vi "HostMain.vi"() -> ()   [LabVIEW 2024]
uses:
  C:/Users/ROAR/Documents/Darren RobUST/grf-mpc-RobUST-trainer/Labview/RobUST_3D_with_Unity_Control_PXI_Low_Level_Only_Streamlined/Vicon_files/ViconDataStreamSDK_DotNET.dll
  Vicon_files/ViconDataStreamSDK_DotNET.dll
  typeDef/Modes_knees.ctl
  <vilib>/Platform/TimedLoop/XDataNode/timing_clust.ctl
  <vilib>/Platform/TimedLoop/XDataNode/nitl_modes.ctl
  <vilib>/Platform/TimedLoop/XDataNode/wakeup.ctl
  <vilib>/Utility/file.llb/Read Delimited Spreadsheet (DBL).vi
  <vilib>/platform/TimedLoop/XDataNode/XDataNode.xnode
  <vilib>/Utility/Variable/NI_VariableUtilities.lvlib
  <vilib>/Platform/TimedLoop/XDataNode/XDNodeRunTimeDep.lvlib
  <vilib>/Analysis/NI_AALBase.lvlib
panel:
  out "listener ID":refnum<k5>
  out "Tokenized Unity Message":string[](array[string])
  out "All tensions mean":dbl[](array[numeric])
  out "Captured tensions mean":dbl[](array[numeric])
  out "Captured tensions standard dev":dbl[](array[numeric])
  in  "Capture current tension mean and standard dev":bool
  out "All tensions standard dev":dbl[](array[numeric])
  out "All tensions history":dbl[][](array[numeric])
  in  "ConstantModeActiveMotorFlags":bool[](array[boolean])
  out "StartManualTensionRecordTimeInSeconds":dbl
  out "RecordTime (s)":dbl
  out "Manually record tensions flag previous state":bool
  in  "MaxTensionsRecordTimeInSecs":dbl
  in  "RecordTensionsForGivenTimeFlag":bool
  out "Task has ended flag":bool
  out "Tension tare values":dbl[](array[numeric])
  in  "Live plot tensions flag":bool
  out "New info string received":bool
  out "Unity task info string":string
  in  "Use sinusoid":bool
  in  "Sinusoid period (s)":dbl
  in  "Sinusoid amplitude (N)":dbl
  in  "Single motor number":i32
  in  "Single motor tension current set value":dbl=10.0 min=10.0
  in  "Single motor tension desired set value":dbl
  in  "Change constant tension value toggle":bool
  out "Finished Late? [i-1]":bool
  out "CablesTared?":bool
  out "Data to save":dbl[][](array[numeric])
  out "Current save file out":path
  out "Connected to Unity last save call?":bool
  in  "Constant mode cable tensions N":dbl
  out "Last Vicon Frame Read":u32
  out "LastTimeUnityTensionsReceivedInMs":u32
  out "TensionsUpdateRateHz":dbl
  out "UnityDesiredCableTensionsInAscendingOrder":dbl[](array[numeric])
  in  "Mode Robot":T1(radio)
  in  "Total Number Motors":i32
  out "Latest tensions":dbl[](array[numeric])
  in  "Tare":bool
  out "Trunk Structure Matrix":dbl[][](array[numeric])
  out "Trunk FF type specifier":string
  out "Center point for FF":dbl[](array[numeric])
  out "Excursion distances Vicon frame":dbl[](array[numeric])
  out "TCP connection to Unity?":bool
  out "Unity TCP connection ID":refnum<k5>
  out "Control point position coords":dbl[](array[numeric])
  in  "Control point data source":T2(radio)
  in  "perturbation directions":string
  in  "Refresh Center 2":bool
  in  "Insert Test Name":string
  out "CurrentPttrunk":cluster{dbl[], dbl[]}
  out "Centertrunk":cluster{dbl[], dbl[]}
  out "xyboundstrunk":cluster{dbl[], dbl[]}
  out "trunk markers":dbl[](array[numeric])
  out "pel markers":dbl[](array[numeric])
  out "whichMode 3":bool[](array[boolean])
  in  "Mode Knees":T3
  out "whichMode 2":bool[](array[boolean])
  in  "?":enum32{"Trunk FF", "Pelvis FF"}(tab)
  in  "Turn On":bool
  out "Trunk Graph":cluster{dbl[], dbl[]}[](graph)
  out "Pelvis Graph":cluster{dbl[], dbl[]}[](graph)
  in  "Turn On Pelv":bool
  out "PelvisGraphyz":cluster{dbl[], dbl[]}[](graph)
  in  "?":T4(tab)
  in  "% Body Weight":dbl=10.0
  in  "FM --- FF":dbl[](array[numeric])=[30.0, 15.0, 15.0, 15.0, 2.0, 2.0]
  in  "Force Field Radius (m)":dbl=0.05
  in  "Update R or FF":bool
  in  "Refresh Center":bool
  in  "Select File with Trunk\nBoundary Points":path=path "" caption="start path"
  in  "Pert Reset":bool
  in  "Apply Pert":bool
  out "Weight [lbs]":dbl
  in  "Update Pert Parameters":bool
  in  "Pert Direction":i16(knob) scale=0.0..7.0
  in  "Rise Time":dbl
  in  "Constant Time":dbl
  in  "Fall Time":dbl
  in  "Amp [%BW]":dbl
  in  "Weight [Kg]":dbl
  in  "Mode Pelvis":enum32{"Idle", "Constant", "Force", "Pert"}(radio)
  out "Boolean":bool
  out "14":cluster{"[0]":dbl, "[1]":dbl}(graph)
  out "13":cluster{"[0]":dbl, "[1]":dbl}(graph)
  out "12":cluster{"[0]":dbl, "[1]":dbl}(graph)
  out "11":cluster{"[0]":dbl, "[1]":dbl}(graph)
  out "10":cluster{"[0]":dbl, "[1]":dbl}(graph)
  out "9":cluster{"[0]":dbl, "[1]":dbl}(graph)
  in  "?":T5(tab)
  in  "Reset Label":bool
  out "Going Up":bool
  in  "record trajectory":bool
  in  "Weight (Kg) --- FF 2":dbl=50.0
  in  "% Body Weight 2":dbl=10.0
  in  "FM --- FF 2":dbl[](array[numeric])=[30.0, 5.0, 5.0, 5.0, 2.0, 2.0]
  in  "Update R or FF 2":bool
  in  "Pelvis Radius FF":dbl=0.03
  in  "Weight [Kg] 3":dbl=75.0
  in  "Amp [%BW] 3":dbl=10.0
  in  "Fall Time 2":dbl=200.0
  in  "Constant Time 2":dbl=200.0
  in  "Rise Time 2":dbl=200.0
  in  "Pert Direction 2":i16(knob) scale=0.0..7.0
  in  "Update Pert Parameters 2":bool
  out "Weight [lbs] 3":dbl
  in  "Apply Pert 2":bool
  in  "Pert Reset 2":bool
  in  "Set Unit Force Vector":dbl[](array[numeric])=[0.0, 0.0, -1.0, 15.0, 2.0, 2.0]
  in  "Update_setForces":bool
  in  "Set % Body Weight":dbl=10.0
  in  "Weight (lb)":dbl=50.0
  out "ATI":dbl[](graph)
  in  "ATI UnBias":bool
  in  "ATI Bias":bool
  out "Saving Data":bool
  out "whichMode":bool[](array[boolean])
  in  "pidGains":dbl[][](array[numeric])=[[3.5, 1.7, 3.0000000000000004, 1.7, 1.7, 3.5, 1.7, 1.7, 2.0, 1.7, 1.7, 3.0, 1.7, 3.5], [0.001, 0.003, 0.003, 0.001, 0.001, 0.003, 0.0008, 0.003, 0.001, 0.003, 0.001, 0.003, 0.001, 0.001], [0.0004, 0.0012, 0.0006, 0.0012, 0.0012, 0.0004, 0.0012, 0.0012, 0.0008, 0.0012, 0.0012, 0.0004, 0.0012, 0.0004]]
  in  "SetPID":bool
  out "4":cluster{"[0]":dbl, "[1]":dbl}(graph)
  out "3":cluster{"[0]":dbl, "[1]":dbl}(graph)
  out "2":cluster{"[0]":dbl, "[1]":dbl}(graph)
  out "1":cluster{"[0]":dbl, "[1]":dbl}(graph)
  out "8":cluster{"[0]":dbl, "[1]":dbl}(graph)
  out "7":cluster{"[0]":dbl, "[1]":dbl}(graph)
  out "6":cluster{"[0]":dbl, "[1]":dbl}(graph)
  out "FB n FF O/P(N)":dbl[](graph)
  out "Current Filename":string
  out ".NET Reference out":refnum<k24>
  out "ViconTab":enum32{"Vicon", "no Vicon"}(tab)
  out "Frame Number":dbl format="%.2f"
  out "Subject Name":string
  out "Markers Count":u32
  in  "Connect\nVicon":bool
  in  "Update\nMarkers":bool
  in  "Vicon Static":bool
  in  "Stream Mode":i32(ring) items=["ClientPull", "ClientPullPreFetch", "ServerPush"]
  out "SDK Version":string
  out "Vicon Connected":bool
  out "5":cluster{"[0]":dbl, "[1]":dbl}(graph)
  out "Voltage O/P (V)":dbl[](graph)
  in  "Use ATI":bool
  in  "ATIDAQFT._FTSensor":refnum<k7>
  in  "UseVicon":bool
  out "Loop Durations (uSec)":i64[](array[numeric])
  in  "DataSave":bool
  in  "Stop":bool
  # "Notes on running HostMain.vi\n1.)  Start  HostMain (auto in Unity control point mode, Idle Trunk mode).\n2.) Then start targetController.vi (for now)\n3.) The tension sensors MUST be tared when the trunk is in  Idle mode.\n4.) Live tension sensor plots are directly below this text! (scroll down)"
  # "STAND TRAINER\n                     Software developed by Vineet Vashista (2014), Moiz Khan (2016-19), Tatiana Luna (2019-20)"
  # "Unity Communication Info Panel"
  # "TCP Connection Status"
  # "General Robot Constants\n(Set in code)"
  # "Current Unity task information string"
  # "Pelvis-Planar"
  # "Data received from Unity (old, deprecated, could delete!)"
  # "Key coordinates"
  # "----->"
  # "Tare tension sensors panel\nNOTE: tare only works in \nRobotMode = Idle"
  # "Manually start tension recording\n(Note: auto-start with Unity messages\nis typical)"
  # "Robot control panel"
  # "2                          3                                           4                                  5                                      6                        7                                  8                           9                                    10                               11                            12                              13                                   14"
  # "HAVE TO TARE\nBEFORE ROBOT\nMODES BECOME\nENABLED!"
  # "Excursion distance measurements"
  # "Constant mode control"
  # "Single motor mode step change"
  # "Motor 1"
  # "Motor 2"
  # "Motor 3"
  # "Motor 4"
  # "Motor 5"
  # "Motor 6"
  # "Motor 7"
  # "Motor 8"
  # "Motor 9"
  # "FF mode type specifier"
  # "Motor 10"
  # "Types: \"I\" = idle; \"B\" = excursion \nboundary 2D"
  # "Motor 11"
  # "Motor 12"
  # "Motor 13"
  # "Motor 14"
  # "PELVIS TOP MOTORS"
  # "TRUNK MOTOR CABLE \nTENSIONS [N]"
  # "Sensor ID: FT5769"
  # "Mx(Nm)"
  # "My(Nm)"
  # "Mz(Nm)"
  # "PID                   QP                  File"
  # "This can be changed only starting of host"
  # "Pelvis-Moments"
  # "PELVIS BOTTOM MOTORS"
  # "SHANK MOTOR CABLE TENSIONS [N]"
  # "Circular Force Field"
  # "Irregular Force Field"
  # "Fz\nMx\nMy\nMz"
  # "30,15,15,15"
  # "Pert Parameters"
  # "FIRST PERT GIVEN BY\nCLICKING TURN ON PERT!!!"
  # "Pert Parameters"
  # "FIRST PERT GIVEN BY\nCLICKING TURN ON PERT!!!"
  # "X\n\nY\n\nZ"
  # "Trunk Static"
  # "Pelvis Static"
  # "Set Tension = Mag + Constant Tension + Step"
  # "TRUNK CONTROL"
  # "PELVIS CONTROL"
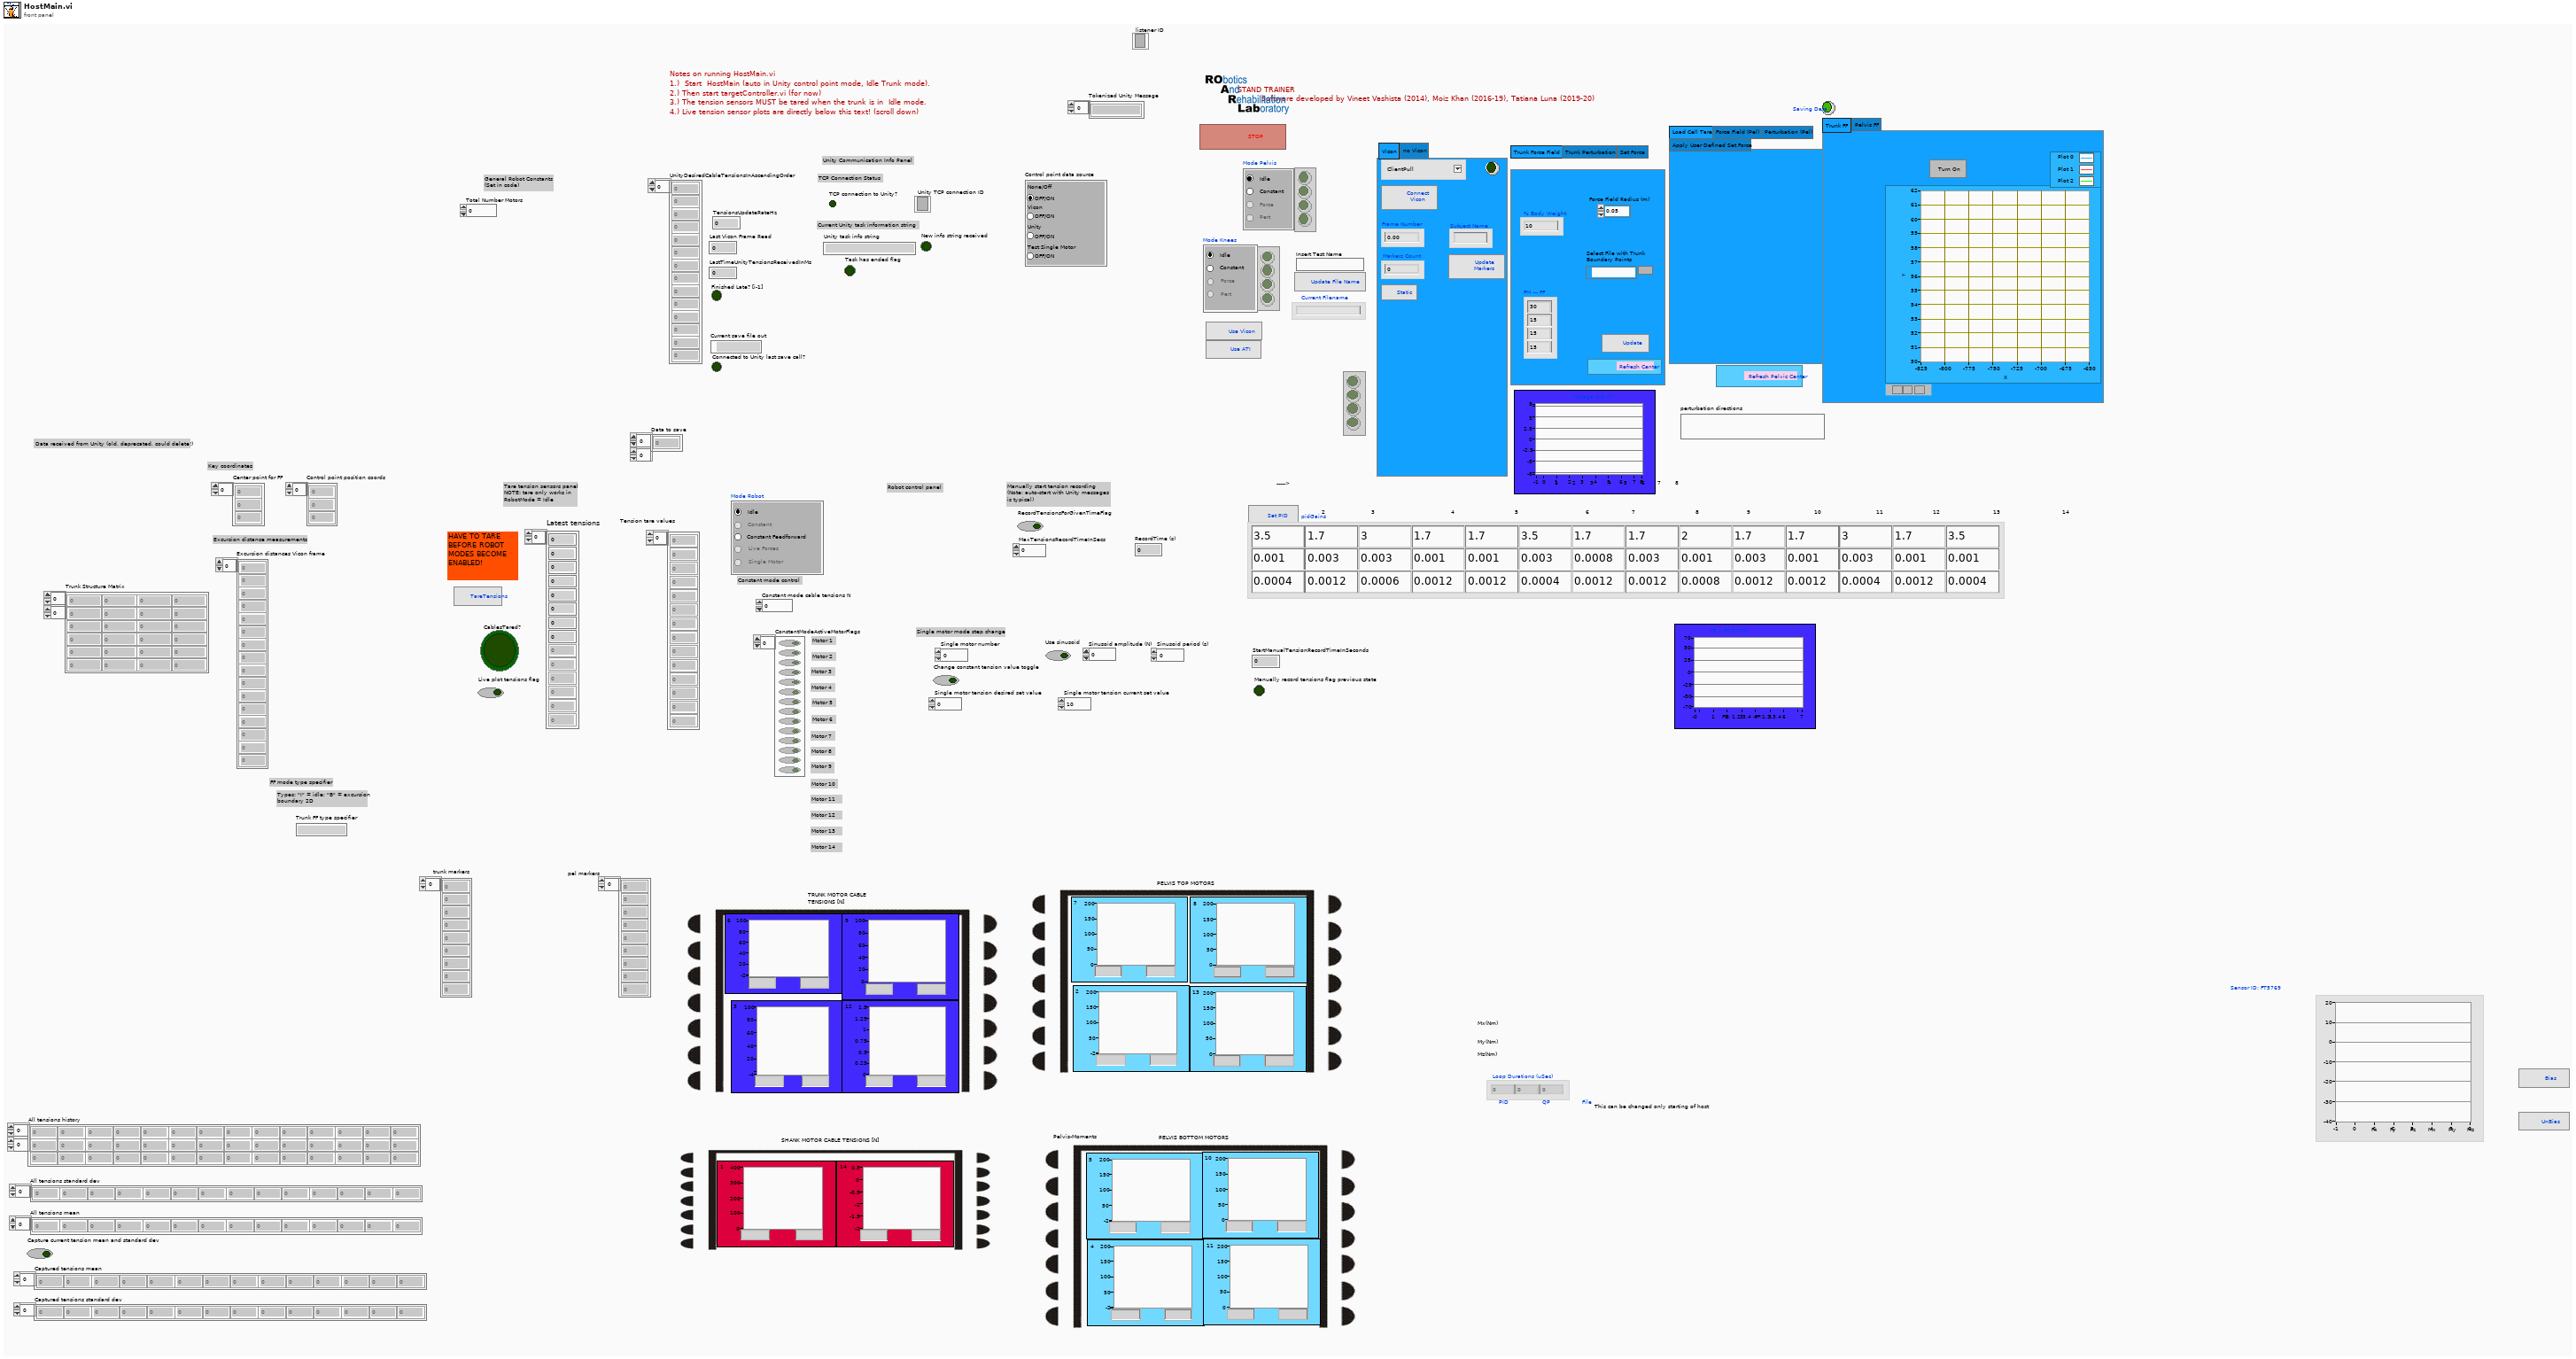
[diagram p1: front panel]
types:
  T1 = enum32{"Idle", "Constant", "Live Forces", "Single Motor", "Constant Feedforward"}
  T2 = enum32{"None/Off", "Vicon", "Unity", "Test Single Motor"}
  T3 = typedef "Modes_knees.ctl" = enum32{"Idle", "Constant", "Force", "Pert"}
  T4 = enum32{"Trunk Force Field", "Trunk Perturbation", "Set Force"}
  T5 = enum32{"Load Cell Tare", "Force Field (Pel)", "Perturbation (Pel)", "Apply User Defined Set Force"}
  T6 = enum32{"Idle", "Constant", "Live Forces", "Single Motor"}
  T7 = enum8{"Enabled", "Disabled", "Disabled and Grayed Out"}
  T8 = typedef "XDNodeRunTimeDep.lvlib/timing_clust.ctl" = cluster{"Expected End [f-1]":u64, "Actual End [f-1]":u64, "Finished Late? [f-1]":bool, "Expected End [i-1]":u64, "Actual End [i-1]":u64, "Finished Late? [i-1]":bool, "Expected Start [i]":u64, "Actual Start [i]":u64, "Expected Start [f]":u64, "Actual Start [f]":u64, "Source Name":string, "Structure Name":string, "Period":i64, "Deadline":i64, "Offset":i64, "Start":i64, "Priority":i32, "Timeout":i32, "Mode":T9, "Wakeup Reason":T10, "Error":errorcluster, "Source Type":string, "Secondary Source Type":string, "Global End Time":u64, "Global Start Time":u64, "Frame Duration":u64, "Iteration Duration":u64, "Assigned CPU":i32, "I/O Scan Engine Mode":u32}
  T9 = typedef "XDNodeRunTimeDep.lvlib/nitl_modes.ctl" = enum32{"No Change", "Process missed periods, maintain original phase", "Discard missed periods, maintain original phase", "Process missed periods, ignore original phase", "Discard missed periods, ignore original phase"}
  T10 = typedef "XDNodeRunTimeDep.lvlib/wakeup.ctl" = enum32{"Normal", "Aborted", "Asynchronous wakeup", "Timing source error", "Timed loop error", "Timeout"}
  T11 = enum16{"Standard", "Buffered", "CRLF", "Immediate"}
  T12 = cluster{"Most Recent Vicon Frame Number":u32, "Corresponding motor tensions":dbl[], "Motor numbers":i32[]}
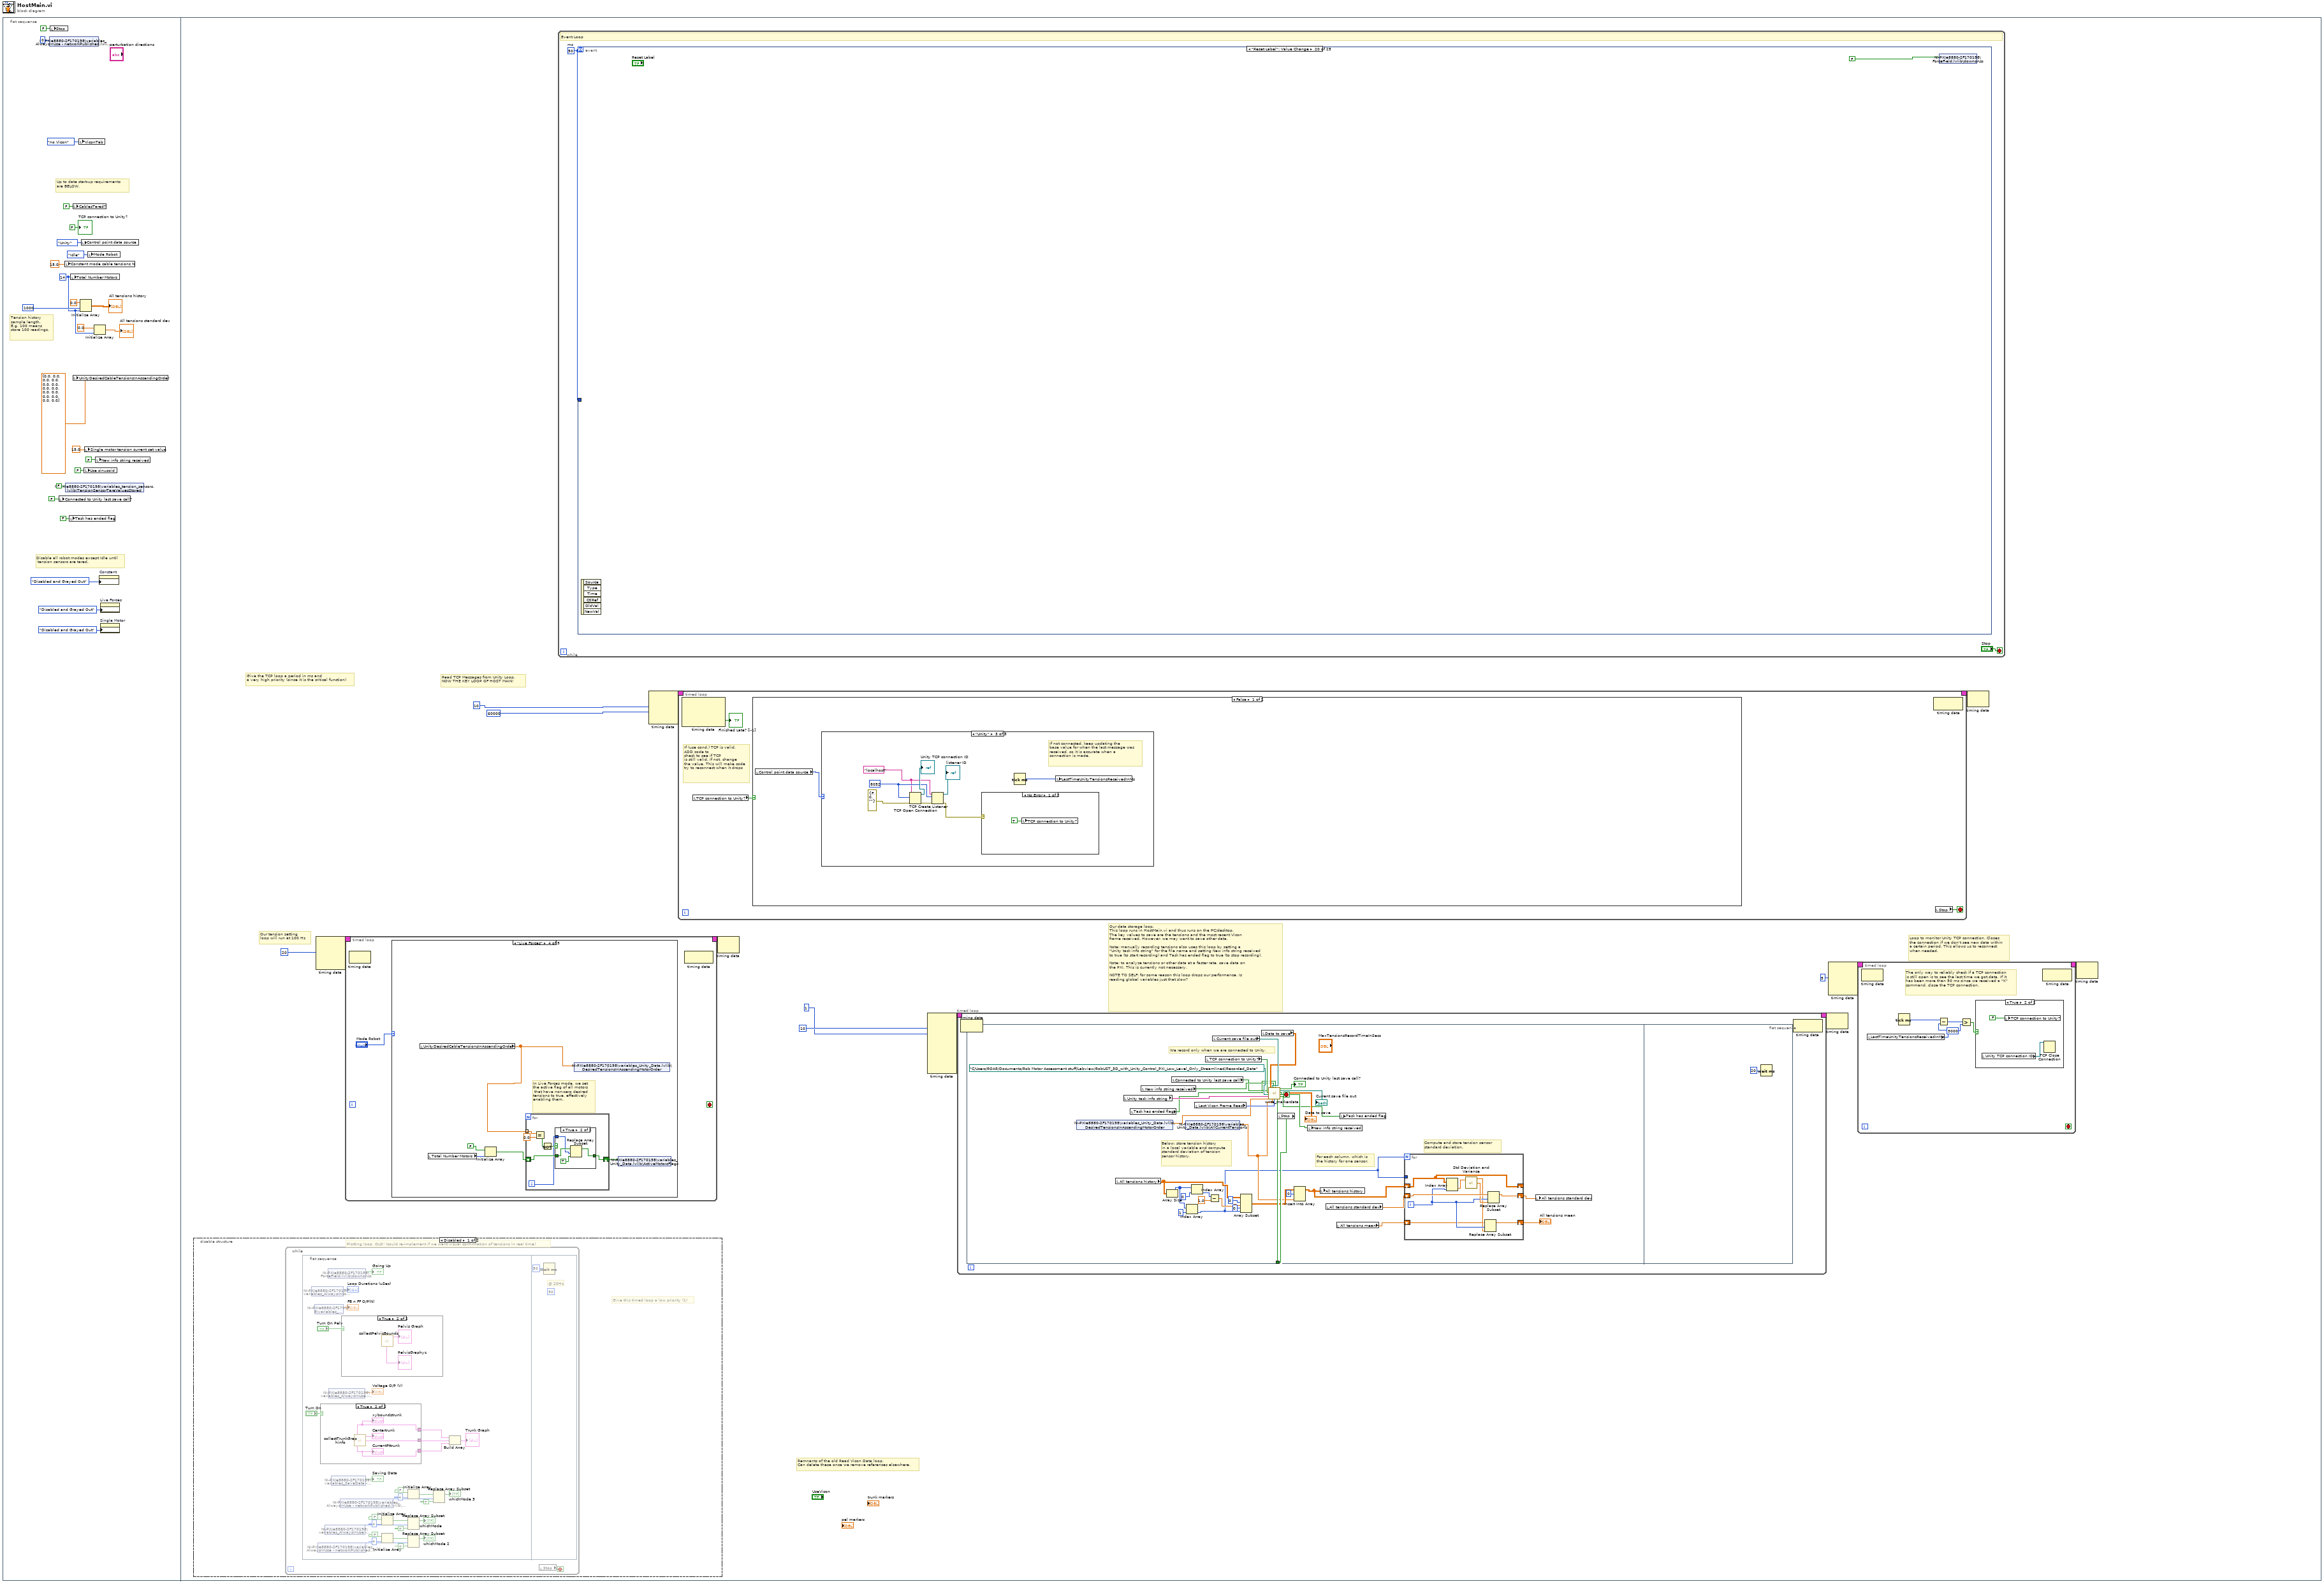
[diagram p0: block diagram]
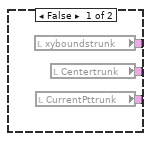
[diagram p3: hidden frame]
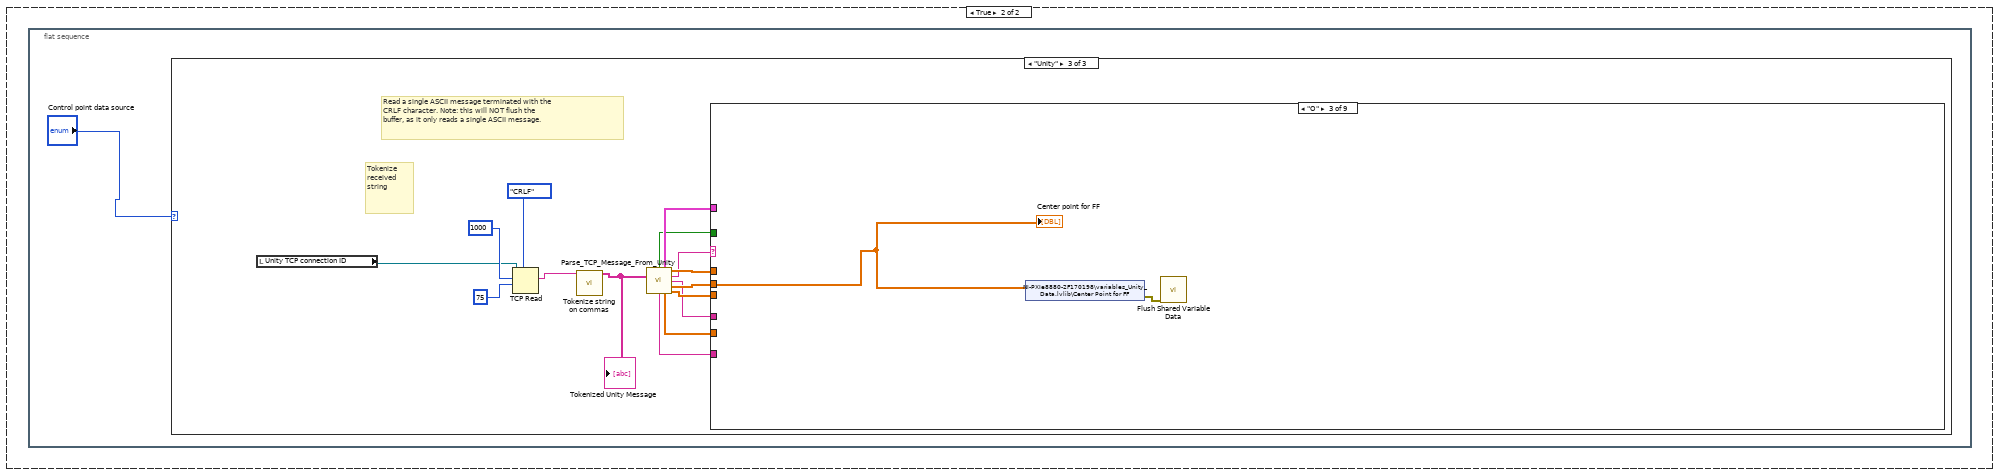
[diagram p9: hidden frame]
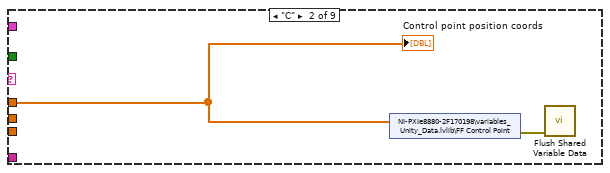
[diagram p13: hidden frame]
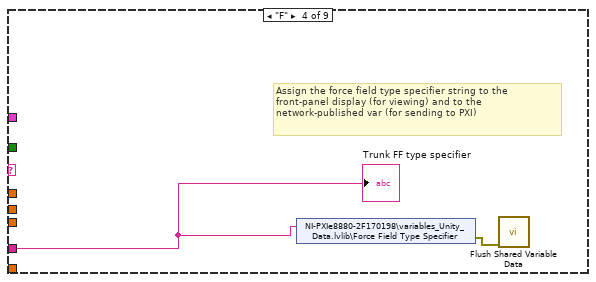
[diagram p14: hidden frame]
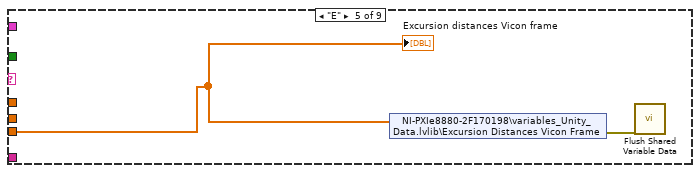
[diagram p15: hidden frame]
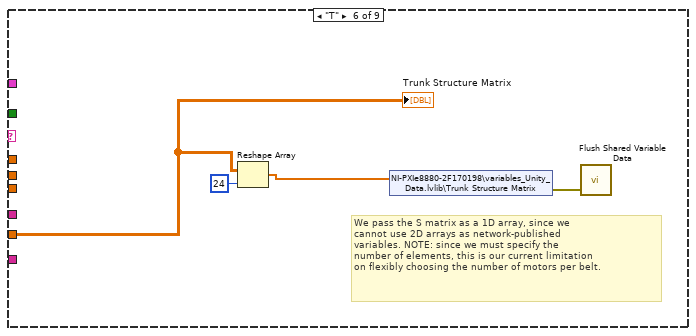
[diagram p16: hidden frame]
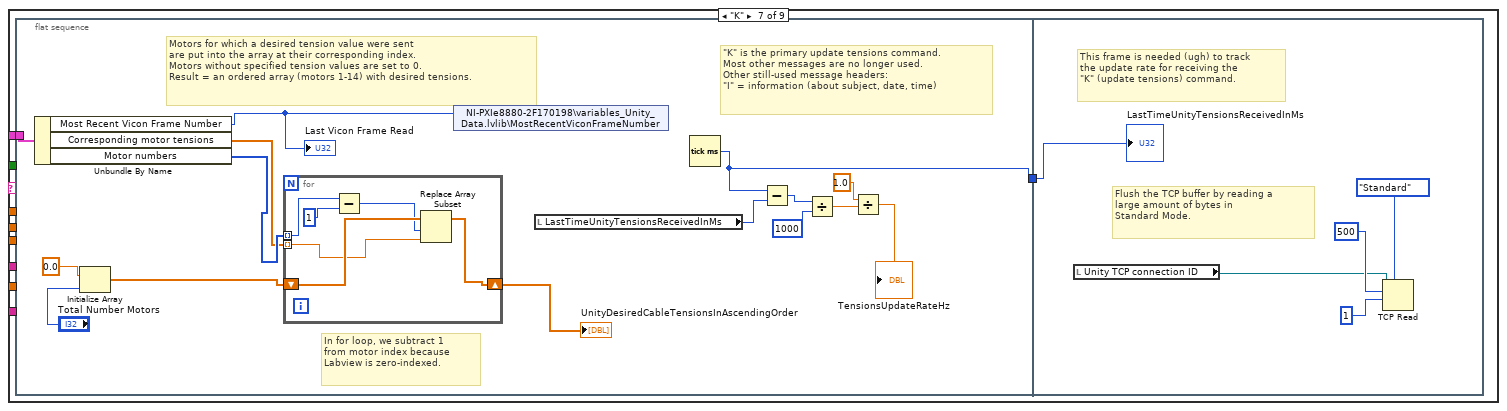
[diagram p17: hidden frame]
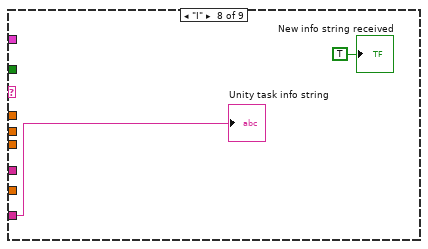
[diagram p18: hidden frame]
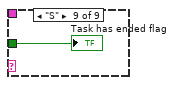
[diagram p19: hidden frame]
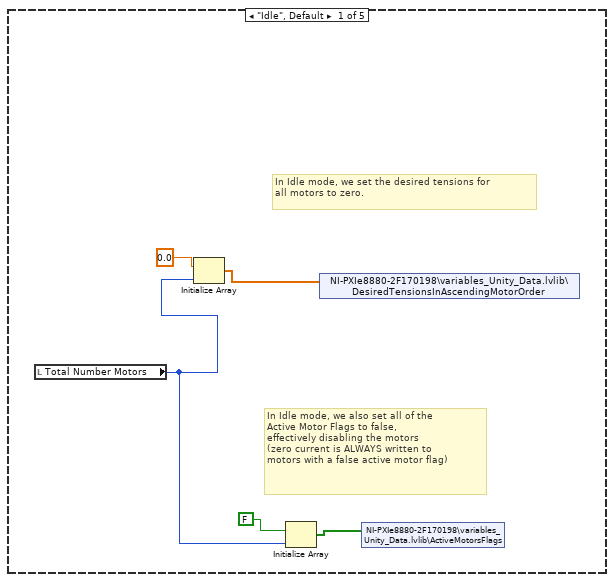
[diagram p20: hidden frame]
diagram:
  n1 = flat-sequence {
    frame #0 {
      w3 = 14 ("Total Number Motors")
      # "Tension history \nsample length. \nE.g. 100 means \nstore 100 readings."
      # "Disable all robot modes except Idle until\n tension sensors are tared."
      # "Up to date start-up requirements\nare BELOW."
      n2 = shared-variable "NI-PXIe8880-2F170198\\variables_AlwaysInUse - networkPublished.lvlib\\Trunk Belt Mode"(i16 0 ("Mode")) -> ()  [unwired: 1 in, 1 out]
      n3 = local write "Stop"(FALSE ("Force")) -> ()
      n4 = local write "Connected to Unity last save call?"(FALSE ("Connected to Unity last save call?")) -> ()
      n5 = local write "Constant mode cable tensions N"(15.0 ("Constant mode cable tensions (N)")) -> ()
      n6 = shared-variable "NI-PXIe8880-2F170198\\variables_tension_sensors.lvlib\\TensionSensorTareValuesStored"(FALSE ("TensionSensorTareValuesStored")) -> ()  [unwired: 1 in, 1 out]
      n7 = local write "Task has ended flag"(FALSE ("Task has ended flag")) -> ()
      n8 = local write "Total Number Motors"(w3) -> ()
      n9 = local write "CablesTared?"(FALSE ("CablesTared?")) -> ()
      n10 = local write "UnityDesiredCableTensionsInAscendingOrder"(dbl[] [0.0, 0.0, 0.0, 0.0, 0.0, 0.0, 0.0, 0.0, 0.0, 0.0, 0.0, 0.0, 0.0, 0.0] ("UnityDesiredCableTensionsInAscendingOrder")) -> ()
      n11 = local write "ViconTab"(enum32{"Vicon", "no Vicon"}."no Vicon" ("ViconTab")) -> ()
      n12 = Initialize Array(0.0 ("element"), 1000 ("dimension size"), w3) -> (→"All tensions history":dbl[][])
      n13 = local write "Control point data source"(enum32{"None/Off", "Vicon", "Unity"}."Unity" ("Control point data source")) -> ()
      n14 = local write "Use sinusoid"(FALSE ("Use sinusoid")) -> ()
      n15 = local write "Single motor tension current set value"(15.0 ("Single motor tension current set value")) -> ()
      n16 = local write "Mode Robot"(T6."Idle" ("Mode Robot")) -> ()
      n17 = Initialize Array(0.0 ("element"), w3) -> (→"All tensions standard dev":dbl[])
      n18 = local write "New info string received"(FALSE ("New info string received")) -> ()
      n19 = property on="Constant" class="Bool (strict)"("DisabledEnum"=T7."Disabled and Grayed Out" ("Disabled")) -> ()  [unwired: 2 in, 2 out]
      n20 = property on="Live Forces" class="Bool (strict)"("DisabledEnum"=T7."Disabled and Grayed Out" ("Disabled")) -> ()  [unwired: 2 in, 2 out]
      n21 = property on="Single Motor" class="Bool (strict)"("DisabledEnum"=T7."Disabled and Grayed Out" ("Disabled")) -> ()  [unwired: 2 in, 2 out]
      "TCP connection to Unity?" <- FALSE ("TCP connection to Unity?")
    }
    frame #1 {
      # "Our data storage loop. \nThis loop runs in HostMain.vi and thus runs on the PC/desktop. \nThe key values to save are the tensions and the most recent Vicon \nframe received. However, we may want to save other data.\n\nNote: manually recording tensions also uses this loop by setting a \n\"Unity task info string\" for the file name and setting New info string received\nto true (to start recording) and Task has ended flag to true (to stop recording). \n\nNote: to analyze tensions or other data at a faster rate, save data on \nthe PXI. This is currently not necessary.\n\nNOTE TO SELF: for some reason this loop drops our performance. Is\nreading global variables just that slow?"
      # "Loop to monitor Unity TCP connection. Closes\nthe connection if we don't see new data within\na certain period. This allows us to reconnect \nwhen needed."
      # "Remnants of the old Read Vicon Data loop. \nCan delete these once we remove references elsewhere."
      # "Give the TCP loop a period in ms and \na very high priority (since it is the critical function)"
      # "Our tension setting\nloop will run at 100 Hz"
      # "Read TCP Messages from Unity Loop. \nNOW THE KEY LOOP OF HOST MAIN!"
      n22 = disable-structure shown="Disabled" {
        frame Disabled {
          # "Give this timed loop a low priority (1)"
          # "Plotting loop. OLD! (could re-implement if we want visual confirmation of tensions in real time)"
          n23 = while {
            stop <- w91 stop-if-true
            n24 = flat-sequence {
              frame #0 {
                n25 = shared-variable "NI-PXIe8880-2F170198\\variables_AlwaysInUse - networkPublished.lvlib\\timings"() -> (→"Loop Durations (uSec)":i64[])  [unwired: 1 in, 1 out]
                n26 = shared-variable "NI-PXIe8880-2F170198\\variables_AlwaysInUse - networkPublished.lvlib\\FBnFF"() -> (→"FB n FF O/P(N)":dbl[])  [unwired: 1 in, 1 out]
                n27 = shared-variable "NI-PXIe8880-2F170198\\variables_AlwaysInUse - networkPublished.lvlib\\whichMode_pel"() -> (w105:i16)  [unwired: 1 in, 1 out]
                n28 = case shown="True" "Turn On" {
                  tunnel: [w125 w128] -> w97
                  tunnel: [w124 w127] -> w96
                  tunnel: [w123 w126] -> w95
                  frame False {
                    n29 = local read "xyboundstrunk"() -> (w125:cluster{dbl[], dbl[]})
                    n30 = local read "CurrentPttrunk"() -> (w123:cluster{dbl[], dbl[]})
                    n31 = local read "Centertrunk"() -> (w124:cluster{dbl[], dbl[]})
                  }
                  frame True {
                    n32 = call "collectTrunkGraphinfo.vi"() -> ("CurrentPttrunk"=w126:cluster{dbl[], dbl[]}, "Centertrunk"=w127:cluster{dbl[], dbl[]}, "xyboundstrunk"=w128:cluster{dbl[], dbl[]})  [unwired: 3 in]
                    "xyboundstrunk" <- w128
                    "Centertrunk" <- w127
                    "CurrentPttrunk" <- w126
                  }
                }
                n33 = shared-variable "NI-PXIe8880-2F170198\\variables_AlwaysInUse - networkPublished.lvlib\\whichMode"() -> (w118:i16)  [unwired: 1 in, 1 out]
                n34 = shared-variable "NI-PXIe8880-2F170198\\ForceField.lvlib\\downorUp"() -> (→"Going Up":bool)  [unwired: 1 in, 1 out]
                n35 = shared-variable "NI-PXIe8880-2F170198\\variables_AlwaysInUse - networkPublished.lvlib\\op2Motor"() -> (→"Voltage O/P (V)":dbl[])  [unwired: 1 in, 1 out]
                n36 = shared-variable "NI-PXIe8880-2F170198\\variables_SaveData - networkPublished.lvlib\\SaveData"() -> (→"Saving Data":bool)  [unwired: 1 in, 1 out]
                n37 = shared-variable "NI-PXIe8880-2F170198\\variables_AlwaysInUse - networkPublished.lvlib\\whichMode_knees"() -> (w103:i16)  [unwired: 1 in, 1 out]
                n38 = case shown="True" "Turn On Pelv" {
                  frame False {
                  }
                  frame True {
                    n39 = call "collectPelvicBounds.vi"() -> ("yzgraph array"=→"PelvisGraphyz":cluster{dbl[], dbl[]}[], "xzgraph"=→"Pelvis Graph":cluster{dbl[], dbl[]}[])  [unwired: 10 in]
                  }
                }
                n40 = Initialize Array(FALSE ("Force"), 4 ("dimension size")) -> (w117:bool[])
                n41 = Initialize Array(FALSE ("Force"), 4 ("dimension size")) -> (w109:bool[])
                n42 = Initialize Array(FALSE ("Force"), 4 ("dimension size")) -> (w102:bool[])
                n43 = Replace Array Subset(array=w117, new element=TRUE ("Force"), index=w118) -> (→"whichMode":bool[])
                n44 = Replace Array Subset(array=w109, new element=TRUE ("Force"), index=w105) -> (→"whichMode 2":bool[])
                n45 = Replace Array Subset(array=w102, new element=TRUE ("Force"), index=w103) -> (→"whichMode 3":bool[])
                n46 = Build Array(w97, w96, w95) -> (→"Trunk Graph":cluster{dbl[], dbl[]}[])
              }
              frame #1 {
                (unwired) u32 50 ("milliseconds to wait")
                # "@ 20Hz"
                n47 = Wait (ms)(milliseconds to wait=u32 50) -> ()  [unwired: 1 out]
              }
            }
            n48 = local read "Stop"() -> (w91:bool)
          }
        }
        frame Enabled {
        }
      }
      n49 = node-c288(i64 20 ("Period")) -> (w38:T8)  [unwired: 3 in]
      n50 = timed-loop {
        timing: w38 -> [_]
        timing-out: [_] -> w37
        stop <- _ stop-if-true
        n51 = node-c288() -> ()  [unwired: 1 in, 1 out]
        n52 = case shown="\"Live Forces\"" "Mode Robot" {
          frame "Idle", Default {
            # "In Idle mode, we also set all of the \nActive Motor Flags to false, \neffectively disabling the motors \n(zero current is ALWAYS written to \nmotors with a false active motor flag)"
            # "In Idle mode, we set the desired tensions for\nall motors to zero."
            n53 = local read "Total Number Motors"() -> (w225:i32)
            n54 = Initialize Array(0.0 ("element"), w225) -> (w227:dbl[])
            n55 = Initialize Array(FALSE, w225) -> (w224:bool[])
            n56 = shared-variable "NI-PXIe8880-2F170198\\variables_Unity_Data.lvlib\\DesiredTensionsInAscendingMotorOrder"(w227) -> ()  [unwired: 1 in, 1 out]
            n57 = shared-variable "NI-PXIe8880-2F170198\\variables_Unity_Data.lvlib\\ActiveMotorsFlags"(w224) -> ()  [unwired: 1 in, 1 out]
          }
          frame "Constant" {
            # "In Constant (tension) mode, we set\nthe Active Motor Flags of all selected motors\nto true, effectively enabling them. \nAll other motor currents will be set to \nzero."
            # "In Constant (tension) mode, we set\nthe desired tensions of all selected motors\nto the constant tension value."
            n58 = local read "Total Number Motors"() -> (w233:i32)
            n59 = Initialize Array(0.0 ("element"), w233) -> (w231:dbl[])
            n60 = for {
              tunnel: "ConstantModeActiveMotorFlags" -> [w237] mode=indexing
              shift-right: [w235] -> w230
              shift-left: w231 -> [w236]
              i -> [w234]
              n61 = case shown="True" w237 {
                tunnel: w236 -> [w238 w241]
                tunnel: [w238 w240] -> w235
                tunnel: w234 -> [_ w239]
                frame False {
                }
                frame True {
                  n62 = Replace Array Subset(array=w241, new element="Constant mode cable tensions N", index=w239) -> (w240:dbl[])
                }
              }
            }
            n63 = shared-variable "NI-PXIe8880-2F170198\\variables_Unity_Data.lvlib\\ActiveMotorsFlags"("ConstantModeActiveMotorFlags") -> ()  [unwired: 1 in, 1 out]
            n64 = shared-variable "NI-PXIe8880-2F170198\\variables_Unity_Data.lvlib\\DesiredTensionsInAscendingMotorOrder"(w230) -> ()  [unwired: 1 in, 1 out]
          }
          frame "Constant Feedforward" {
            # "In Constant (tension) mode, we set\nthe Active Motor Flags of all selected motors\nto true, effectively enabling them. \nAll other motor currents will be set to \nzero."
            # "In Constant (tension) mode, we set\nthe desired tensions of all selected motors\nto the constant tension value."
            n65 = local read "ConstantModeActiveMotorFlags"() -> (w243:bool[])
            n66 = local read "Total Number Motors"() -> (w247:i32)
            n67 = Initialize Array(0.0 ("element"), w247) -> (w245:dbl[])
            n68 = for {
              tunnel: w243 -> [w251] mode=indexing
              shift-right: [w249] -> w244
              shift-left: w245 -> [w250]
              i -> [w248]
              n69 = case shown="True" w251 {
                tunnel: w250 -> [w252 w256]
                tunnel: [w252 w255] -> w249
                tunnel: w248 -> [_ w254]
                frame False {
                }
                frame True {
                  n70 = local read "Constant mode cable tensions N"() -> (w253:dbl)
                  n71 = Replace Array Subset(array=w256, new element=w253, index=w254) -> (w255:dbl[])
                }
              }
            }
            n72 = shared-variable "NI-PXIe8880-2F170198\\variables_Unity_Data.lvlib\\ActiveMotorsFlags"(w243) -> ()  [unwired: 1 in, 1 out]
            n73 = shared-variable "NI-PXIe8880-2F170198\\variables_Unity_Data.lvlib\\DesiredTensionsInAscendingMotorOrder"(w244) -> ()  [unwired: 1 in, 1 out]
          }
          frame "Live Forces" {
            # "In Live Forces mode, we set\nthe active flag of all motors\n that have non-zero desired \ntensions to true, effectively\nenabling them."
            n74 = local read "UnityDesiredCableTensionsInAscendingOrder"() -> (w261:dbl[])
            n75 = local read "Total Number Motors"() -> (w260:i32)
            n76 = Initialize Array(FALSE, w260) -> (w258:bool[])
            n77 = for {
              tunnel: w261 -> [w268] mode=indexing
              shift-right: [w263] -> w257
              shift-left: w258 -> [w264]
              i -> [w262]
              n78 = Equal?(x=w268, y=0.0) -> (x = y?=w266:bool)
              n79 = Not(x=w266) -> (.not. x?=w265:bool)
              n80 = case shown="True" w265 {
                tunnel: w264 -> [w269 w273]
                tunnel: [w269 w270] -> w263
                tunnel: w262 -> [_ w271]
                frame False {
                }
                frame True {
                  n81 = Replace Array Subset(array=w273, new element=TRUE ("new element/subarray"), index=w271) -> (w270:bool[])
                }
              }
            }
            n82 = shared-variable "NI-PXIe8880-2F170198\\variables_Unity_Data.lvlib\\DesiredTensionsInAscendingMotorOrder"(w261) -> ()  [unwired: 1 in, 1 out]
            n83 = shared-variable "NI-PXIe8880-2F170198\\variables_Unity_Data.lvlib\\ActiveMotorsFlags"(w257) -> ()  [unwired: 1 in, 1 out]
          }
          frame "Single Motor" {
            # "Only one motor is flagged as \nactive in Single Motor control\nmode. All other motor currents\nwill be set to zero."
            # "Subtract 1 b/c of \nzero-indexing"
            n84 = local read "Total Number Motors"() -> (w279:i32)
            n85 = Subtract(x="Single motor number", y=1) -> (x-y=w276:i32)
            n86 = local read "Tension tare values"() -> (w280:dbl[])
            n87 = Initialize Array(FALSE, w279) -> (w277:bool[])
            n88 = Replace Array Subset(array=w277, new element=TRUE ("new element/subarray"), index=w276) -> (w274:bool[])
            n89 = Replace Array Subset(array=w280, new element="Single motor tension current set value", index=w276) -> (w284:dbl[])
            n90 = shared-variable "NI-PXIe8880-2F170198\\variables_Unity_Data.lvlib\\DesiredTensionsInAscendingMotorOrder"(w284) -> ()  [unwired: 1 in, 1 out]
            n91 = shared-variable "NI-PXIe8880-2F170198\\variables_Unity_Data.lvlib\\ActiveMotorsFlags"(w274) -> ()  [unwired: 1 in, 1 out]
          }
        }
        n92 = node-c288() -> ()  [unwired: 1 in, 1 out]
      }
      n93 = while {
        stop <- "Stop" stop-if-true
        w291 = 50  # ms
        # "Event Loop"
        n94 = event shown="[19] \"Reset Label\": Value Change" {
          selector: _ -> [_ _ _ _ _ _ _ _ _ _ _ _ _ _ _ _ _ _ _ _ _ _ _ _ _]
          dyn-events: _ -> [_ _ _ _ _ _ _ _ _ _ _ _ _ _ _ _ _ _ _ _ _ _ _ _ _]
          timeout: w291 -> [_ _ _ _ _ _ _ _ _ _ _ _ _ _ _ _ _ _ _ _ _ _ _ _ _]
          tunnel: w291 -> [w303 _ _ _ _ _ _ _ _ _ _ _ _ _ _ _ _ _ _ _ _ _ _ _ _]
          event Timeout {
            # "If the button for capturing the current tension standard deviation \nis being pressed, store whatever the current values are. \nUsing a \"switch-until-released\" mechanical action on \nthe capture button means a click will just capture the current values."
            # "This block handles manually recording the cable tensions (usually for single motor testing)"
            # "If we want to \nlive-plot the \ntension values"
            # "This event runs every time the timeout period expires. \nSo, since buttons are rarely pressed, it runs quite often.\nUse this event to update states of variables (e.g. mode \nchanges) in a non-urgent way."
            # "On timeout (every 50 ms, if no button presses), \nupdate the robot mode."
            # "THIS CASE STRUCTURE:\n- Reads ATI F/T data, if \nusing"
            # "THIS CASE STRUCTURE:\n- Allows us to (manually?)\nset the PID gains if desired."
            # "THIS CASE STRUCTURE: \n- Tare tension sensors \nin robot mode \"Idle\" only."
            n95 = event-data() -> ()  [unwired: 1 in, 3 out]
            n96 = local read "Single motor number"() -> (w297:i32)
            n97 = local read "Mode Robot"() -> (w298:T1)
            n98 = disable-structure shown="Disabled" {
              frame Disabled {
              }
              frame Enabled {
              }
            }
            n99 = Divide(x=w303, y=1000.0) -> (x/y=w301:dbl)
            n100 = shared-variable "NI-PXIe8880-2F170198\\variables_Unity_Data.lvlib\\RobotControlModeAsInt"(w298) -> ()  [unwired: 1 in, 1 out]
            n101 = shared-variable "NI-PXIe8880-2F170198\\variables_Unity_Data.lvlib\\SingleMotorControlModeMotorNumber"(w297) -> ()  [unwired: 1 in, 1 out]
            n102 = property class="WFChart (strict)"("XScale.Multiplier"=w301) -> ()  [unwired: 2 in, 2 out]
            n103 = case shown="False" "Use ATI" {
              frame False {
              }
              frame True {
                n104 = shared-variable "NI-PXIe8880-2F170198\\variables_ATI - networkPublished.lvlib\\ATI_FM"() -> (→"ATI":dbl[])  [unwired: 1 in, 1 out]
              }
            }
            n105 = case shown="False" "SetPID" {
              selector: "SetPID" -> [_ w402]
              frame False {
              }
              frame True {
                n106 = shared-variable "NI-PXIe8880-2F170198\\variables_ToSetPID - networkPublished.lvlib\\SetPID"(w402) -> ()  [unwired: 1 in, 1 out]
                n107 = Transpose 2D Array(2D array="pidGains") -> (transposed array=w400:dbl[][])
                n108 = Reshape Array(w400, 42 ("dimension size")) -> (w399:dbl[])
                n109 = shared-variable "NI-PXIe8880-2F170198\\variables_ToSetPID - networkPublished.lvlib\\pidGains"(w399) -> ()  [unwired: 1 in, 1 out]
              }
            }
            n110 = shared-variable "NI-PXIe8880-2F170198\\variables_Unity_Data.lvlib\\DesiredTensionsInAscendingMotorOrder"() -> (w299:dbl[])  [unwired: 1 in, 1 out]
            n111 = shared-variable "NI-PXIe8880-2F170198\\variables_Unity_Data.lvlib\\AllCurrentTensions"() -> (w294:dbl[])  [unwired: 1 in, 1 out]
            "Latest tensions" <- w294
            n112 = local read "Mode Robot"() -> (w304:T1)
            n113 = case shown="\"Idle\", Default" w304 {
              frame "Idle", Default {
                # "Load Cell Tare"
                n114 = shared-variable "NI-PXIe8880-2F170198\\variables_tension_sensors.lvlib\\TensionSensorTareValuesStored"() -> (w404:bool)  [unwired: 1 in, 1 out]
                n115 = case shown="True" "Tare" {
                  selector: "Tare" -> [_ w416]
                  tunnel: [w413 w415] -> w406
                  tunnel: [FALSE w416] -> w405
                  frame False {
                    n116 = local read "Tension tare values"() -> (w413:dbl[])
                  }
                  frame True {
                    n117 = local read "Latest tensions"() -> (w415:dbl[])
                    "Tension tare values" <- w415
                    "Boolean" <- w416
                  }
                }
                n118 = case shown="True" w404 {
                  frame False {
                  }
                  frame True {
                    # "If the PXI has tared\nthe tension sensor values,\nenable other robot modes."
                    n119 = property on="Idle" class="Bool (strict)"("DisabledEnum"=T7."Enabled" ("Disabled")) -> ()  [unwired: 2 in, 2 out]
                    n120 = property on="Constant" class="Bool (strict)"("DisabledEnum"=T7."Enabled" ("Disabled")) -> ()  [unwired: 2 in, 2 out]
                    n121 = property on="Live Forces" class="Bool (strict)"("DisabledEnum"=T7."Enabled" ("Disabled")) -> ()  [unwired: 2 in, 2 out]
                    n122 = property on="Single Motor" class="Bool (strict)"("DisabledEnum"=T7."Enabled" ("Disabled")) -> ()  [unwired: 2 in, 2 out]
                    "CablesTared?" <- TRUE ("CablesTared?")
                  }
                }
                n123 = shared-variable "NI-PXIe8880-2F170198\\Load Cell Tare.lvlib\\TareTrue"(w405) -> ()  [unwired: 1 in, 1 out]
                n124 = shared-variable "NI-PXIe8880-2F170198\\Load Cell Tare.lvlib\\Loadcelltare"(w406) -> ()  [unwired: 1 in, 1 out]
              }
              frame "Constant" {
              }
              frame "Live Forces" {
              }
              frame "Single Motor" {
                n125 = case shown="True" "Use sinusoid" {
                  frame False {
                  }
                  frame True {
                    n126 = local read "Single motor tension desired set value"() -> (w420:dbl)
                    n127 = Multiply(x=2.0, y=3.141592653589793) -> (x*y=w426:dbl)
                    n128 = Tick Count (ms)() -> (millisecond timer value=w429:u32)
                    n129 = Divide(x=w429, y=1000.0) -> (x/y=w427:dbl)
                    n130 = Multiply(x=w426, y=w427) -> (x*y=w425:dbl)
                    n131 = Divide(x=w425, y="Sinusoid period (s)") -> (x/y=w423:dbl)
                    n132 = Cosine(x=w423) -> (cos(x)=w422:dbl)
                    n133 = Multiply(x="Sinusoid amplitude (N)", y=w422) -> (x*y=w419:dbl)
                    n134 = Add(x=w420, y=w419) -> (x+y=w418:dbl)
                    n135 = local write "Single motor tension current set value"(w418) -> ()
                  }
                }
              }
            }
            n136 = case shown="True" "RecordTensionsForGivenTimeFlag" {
              selector: "RecordTensionsForGivenTimeFlag" -> [w316 w335]
              tunnel: [w316 w335] -> w296
              frame True {
                # "If we have recorded tensions for long \nenough, stop the recording by flipping \nthe record state flag to false."
                # "If the current recording state is different than the last state"
                # "In the ManualRecording = true state, \nkeep track of the recording time"
                n137 = local read "Manually record tensions flag previous state"() -> (w318:bool)
                n138 = Not Equal?(x=w316, y=w318) -> (x != y?=w317:bool)
                n139 = case shown="True" w317 {
                  tunnel: [w321 w327] -> w310
                  frame False {
                    n140 = Tick Count (ms)() -> (millisecond timer value=w321:u32)
                  }
                  frame True {
                    # "Create a manual recording file name\nwith hour_minute appended."
                    # "Mark start time of recording."
                    n141 = Tick Count (ms)() -> (millisecond timer value=w327:u32)
                    n142 = Format Date/Time String(time format string (%c)="%I", UTC format=FALSE) -> (date/time string=w331:string)  [unwired: 1 in]
                    n143 = Format Date/Time String(time format string (%c)="%M", UTC format=FALSE) -> (date/time string=w322:string)  [unwired: 1 in]
                    n144 = Divide(x=w327, y=1000.0) -> (x/y=→"StartManualTensionRecordTimeInSeconds":dbl)
                    n145 = Concatenate Strings("Manual_Tension_Record_" ("string"), w331, "_" ("string"), w322) -> (w326:string)
                    n146 = local write "Unity task info string"(w326) -> ()
                    n147 = local write "New info string received"(TRUE ("New info string received")) -> ()
                  }
                }
                n148 = local read "MaxTensionsRecordTimeInSecs"() -> (w312:dbl)
                n149 = local read "StartManualTensionRecordTimeInSeconds"() -> (w315:dbl)
                n150 = Divide(x=w310, y=1000.0) -> (x/y=w313:dbl)
                n151 = Subtract(x=w313, y=w315) -> (x-y=w309:dbl)
                "RecordTime (s)" <- w309
                n152 = Greater Or Equal?(x=w309, y=w312) -> (x >= y?=w311:bool)
                n153 = case shown="True" w311 {
                  frame False {
                  }
                  frame True {
                    n154 = local write "RecordTime (s)"(0.0 ("RecordTime (s)")) -> ()
                    n155 = local write "RecordTensionsForGivenTimeFlag"(FALSE ("RecordTensionsForGivenTimeFlag")) -> ()
                  }
                }
              }
              frame False {
                # "If the current recording state is different than the last state"
                n156 = local read "Manually record tensions flag previous state"() -> (w337:bool)
                n157 = Not Equal?(x=w335, y=w337) -> (x != y?=w336:bool)
                n158 = case shown="True" w336 {
                  frame False {
                  }
                  frame True {
                    # "If the recording flag just got set to false, then \nthe recording has ended."
                    n159 = local write "Task has ended flag"(TRUE ("Task has ended flag")) -> ()
                  }
                }
              }
            }
            "Manually record tensions flag previous state" <- w296
            n160 = case shown="True" "Live plot tensions flag" {
              tunnel: w299 -> [_ w375]
              tunnel: w294 -> [_ w339]
              frame False {
              }
              frame True {
                # "Send the tension data to the waveform plots for all tension sensors."
                n161 = Index Array(array=w339, index #1=0 ("index")) -> (element #1=w372:dbl, element #2=w383:dbl, element #3=w385:dbl, element #4=w387:dbl, element #5=w389:dbl, element #6=w391:dbl, element #7=w393:dbl, element #8=w398:dbl, element #9=w351:dbl, element #10=w349:dbl, element #11=w347:dbl, element #12=w345:dbl, element #13=w343:dbl, element #14=w341:dbl)  [unwired: 13 in]
                n162 = Index Array(array=w375, index #1=0 ("index")) -> (element #1=w373:dbl, element #2=w384:dbl, element #3=w386:dbl, element #4=w388:dbl, element #5=w390:dbl, element #6=w392:dbl, element #7=w394:dbl, element #8=w397:dbl, element #9=w350:dbl, element #10=w348:dbl, element #11=w346:dbl, element #12=w344:dbl, element #13=w342:dbl, element #14=w340:dbl)  [unwired: 13 in]
                n163 = Build Array(w372, w373) -> (w374:dbl[])
                n164 = Build Array(w383, w384) -> (w377:dbl[])
                n165 = Build Array(w385, w386) -> (w378:dbl[])
                n166 = Build Array(w387, w388) -> (w379:dbl[])
                n167 = Build Array(w389, w390) -> (w380:dbl[])
                n168 = Build Array(w391, w392) -> (w381:dbl[])
                n169 = Build Array(w393, w394) -> (w382:dbl[])
                n170 = Build Array(w398, w397) -> (w396:dbl[])
                n171 = Build Array(w351, w350) -> (w363:dbl[])
                n172 = Build Array(w349, w348) -> (w361:dbl[])
                n173 = Build Array(w347, w346) -> (w359:dbl[])
                n174 = Build Array(w345, w344) -> (w357:dbl[])
                n175 = Build Array(w343, w342) -> (w355:dbl[])
                n176 = Build Array(w341, w340) -> (w353:dbl[])
                n177 = Array To Cluster(array=w374) -> (cluster=→"1":cluster{"[0]":dbl, "[1]":dbl})
                n178 = Array To Cluster(array=w377) -> (cluster=→"2":cluster{"[0]":dbl, "[1]":dbl})
                n179 = Array To Cluster(array=w378) -> (cluster=→"3":cluster{"[0]":dbl, "[1]":dbl})
                n180 = Array To Cluster(array=w379) -> (cluster=→"4":cluster{"[0]":dbl, "[1]":dbl})
                n181 = Array To Cluster(array=w380) -> (cluster=→"5":cluster{"[0]":dbl, "[1]":dbl})
                n182 = Array To Cluster(array=w381) -> (cluster=→"6":cluster{"[0]":dbl, "[1]":dbl})
                n183 = Array To Cluster(array=w382) -> (cluster=→"7":cluster{"[0]":dbl, "[1]":dbl})
                n184 = Array To Cluster(array=w396) -> (cluster=→"8":cluster{"[0]":dbl, "[1]":dbl})
                n185 = Array To Cluster(array=w363) -> (cluster=→"9":cluster{"[0]":dbl, "[1]":dbl})
                n186 = Array To Cluster(array=w361) -> (cluster=→"10":cluster{"[0]":dbl, "[1]":dbl})
                n187 = Array To Cluster(array=w359) -> (cluster=→"11":cluster{"[0]":dbl, "[1]":dbl})
                n188 = Array To Cluster(array=w357) -> (cluster=→"12":cluster{"[0]":dbl, "[1]":dbl})
                n189 = Array To Cluster(array=w355) -> (cluster=→"13":cluster{"[0]":dbl, "[1]":dbl})
                n190 = Array To Cluster(array=w353) -> (cluster=→"14":cluster{"[0]":dbl, "[1]":dbl})
              }
            }
            n191 = case shown="True" "Capture current tension mean and standard dev" {
              frame False {
              }
              frame True {
                n192 = local read "All tensions standard dev"() -> (→"Captured tensions standard dev":dbl[])
                n193 = local read "All tensions mean"() -> (→"Captured tensions mean":dbl[])
              }
            }
          }
          event "Change constant tension value toggle": Value Change {
            n194 = event-data() -> ()  [unwired: 1 in, 6 out]
            n195 = local write "Single motor tension current set value"("Single motor tension desired set value") -> ()
          }
          event "Mode Pelvis": Value Change {
            n196 = event-data() -> ("NewVal"=w435:enum32{"Idle", "Constant", "Force", "Pert"})  [unwired: 1 in, 5 out]
            n197 = case shown="\"Pert\"" w435 {
              tunnel: [i16 0 ("Mode") i16 1 ("Mode") i16 2 ("Mode") i16 3 ("Mode")] -> w434
              frame "Idle", Default {
                n198 = property on="Mode Pelvis" class="RadioBtnsControl (strict)"() -> ("Controls[]"=w436:refnum<vi>[])  [unwired: 2 in, 2 out]
                n199 = Index Array(array=w436, index #1=1 ("index")) -> (element #1=w444:refnum<vi>, element #2=w438:refnum<vi>, element #3=w439:refnum<vi>)  [unwired: 2 in]
                n200 = property class="Ctl"(reference=w444, "DisabledEnum"=T7."Enabled" ("Disabled")) -> ()  [unwired: 1 in, 2 out]
                n201 = property class="Ctl"(reference=w438, "DisabledEnum"=T7."Disabled and Grayed Out" ("Disabled")) -> ()  [unwired: 1 in, 2 out]
                n202 = property class="Ctl"(reference=w439, "DisabledEnum"=T7."Disabled and Grayed Out" ("Disabled")) -> ()  [unwired: 1 in, 2 out]
              }
              frame "Constant" {
                n203 = property on="Mode Pelvis" class="RadioBtnsControl (strict)"() -> ("Controls[]"=w445:refnum<vi>[])  [unwired: 2 in, 2 out]
                n204 = Index Array(array=w445, index #1=0 ("index"), index #2=2 ("index"), index #3=3 ("index")) -> (element #1=w455:refnum<vi>, element #2=w447:refnum<vi>, element #3=w448:refnum<vi>)
                n205 = property class="Ctl"(reference=w455, "DisabledEnum"=T7."Enabled" ("Disabled")) -> ()  [unwired: 1 in, 2 out]
                n206 = property class="Ctl"(reference=w447, "DisabledEnum"=T7."Enabled" ("Disabled")) -> ()  [unwired: 1 in, 2 out]
                n207 = property class="Ctl"(reference=w448, "DisabledEnum"=T7."Enabled" ("Disabled")) -> ()  [unwired: 1 in, 2 out]
              }
              frame "Force" {
                n208 = property on="Mode Pelvis" class="RadioBtnsControl (strict)"() -> ("Controls[]"=w456:refnum<vi>[])  [unwired: 2 in, 2 out]
                n209 = Index Array(array=w456, index #1=0 ("index"), index #2=1 ("index"), index #3=3 ("index")) -> (element #1=w466:refnum<vi>, element #2=w458:refnum<vi>, element #3=w459:refnum<vi>)
                n210 = property class="Ctl"(reference=w466, "DisabledEnum"=T7."Disabled and Grayed Out" ("Disabled")) -> ()  [unwired: 1 in, 2 out]
                n211 = property class="Ctl"(reference=w458, "DisabledEnum"=T7."Enabled" ("Disabled")) -> ()  [unwired: 1 in, 2 out]
                n212 = property class="Ctl"(reference=w459, "DisabledEnum"=T7."Disabled and Grayed Out" ("Disabled")) -> ()  [unwired: 1 in, 2 out]
              }
              frame "Pert" {
                n213 = property on="Mode Pelvis" class="RadioBtnsControl (strict)"() -> ("Controls[]"=w467:refnum<vi>[])  [unwired: 2 in, 2 out]
                n214 = Index Array(array=w467, index #1=0 ("index"), index #2=1 ("index"), index #3=2 ("index")) -> (element #1=w477:refnum<vi>, element #2=w469:refnum<vi>, element #3=w470:refnum<vi>)
                n215 = property class="Ctl"(reference=w477, "DisabledEnum"=T7."Disabled and Grayed Out" ("Disabled")) -> ()  [unwired: 1 in, 2 out]
                n216 = property class="Ctl"(reference=w469, "DisabledEnum"=T7."Enabled" ("Disabled")) -> ()  [unwired: 1 in, 2 out]
                n217 = property class="Ctl"(reference=w470, "DisabledEnum"=T7."Disabled and Grayed Out" ("Disabled")) -> ()  [unwired: 1 in, 2 out]
              }
            }
            n218 = shared-variable "NI-PXIe8880-2F170198\\variables_AlwaysInUse - networkPublished.lvlib\\Mode_pelvis"(w434) -> ()  [unwired: 1 in, 1 out]
          }
          event Value Change {
            n219 = event-data() -> ("NewVal"=w479:T3)  [unwired: 1 in, 5 out]
            n220 = case shown="\"Pert\"" w479 {
              tunnel: [i16 0 ("Mode") i16 1 ("Mode") i16 2 ("Mode") i16 3 ("Mode")] -> w478
              frame "Idle", Default {
                n221 = property on="Mode Knees" class="RadioBtnsControl (strict)"() -> ("Controls[]"=w480:refnum<vi>[])  [unwired: 2 in, 2 out]
                n222 = Index Array(array=w480, index #1=1 ("index")) -> (element #1=w488:refnum<vi>, element #2=w482:refnum<vi>, element #3=w483:refnum<vi>)  [unwired: 2 in]
                n223 = property class="Ctl"(reference=w488, "DisabledEnum"=T7."Enabled" ("Disabled")) -> ()  [unwired: 1 in, 2 out]
                n224 = property class="Ctl"(reference=w482, "DisabledEnum"=T7."Disabled and Grayed Out" ("Disabled")) -> ()  [unwired: 1 in, 2 out]
                n225 = property class="Ctl"(reference=w483, "DisabledEnum"=T7."Disabled and Grayed Out" ("Disabled")) -> ()  [unwired: 1 in, 2 out]
              }
              frame "Constant" {
                n226 = property on="Mode Knees" class="RadioBtnsControl (strict)"() -> ("Controls[]"=w489:refnum<vi>[])  [unwired: 2 in, 2 out]
                n227 = Index Array(array=w489, index #1=0 ("index"), index #2=2 ("index"), index #3=3 ("index")) -> (element #1=w499:refnum<vi>, element #2=w491:refnum<vi>, element #3=w492:refnum<vi>)
                n228 = property class="Ctl"(reference=w499, "DisabledEnum"=T7."Enabled" ("Disabled")) -> ()  [unwired: 1 in, 2 out]
                n229 = property class="Ctl"(reference=w491, "DisabledEnum"=T7."Enabled" ("Disabled")) -> ()  [unwired: 1 in, 2 out]
                n230 = property class="Ctl"(reference=w492, "DisabledEnum"=T7."Enabled" ("Disabled")) -> ()  [unwired: 1 in, 2 out]
              }
              frame "Force" {
                n231 = property on="Mode Knees" class="RadioBtnsControl (strict)"() -> ("Controls[]"=w500:refnum<vi>[])  [unwired: 2 in, 2 out]
                n232 = Index Array(array=w500, index #1=0 ("index"), index #2=1 ("index"), index #3=3 ("index")) -> (element #1=w510:refnum<vi>, element #2=w502:refnum<vi>, element #3=w503:refnum<vi>)
                n233 = property class="Ctl"(reference=w510, "DisabledEnum"=T7."Disabled and Grayed Out" ("Disabled")) -> ()  [unwired: 1 in, 2 out]
                n234 = property class="Ctl"(reference=w502, "DisabledEnum"=T7."Enabled" ("Disabled")) -> ()  [unwired: 1 in, 2 out]
                n235 = property class="Ctl"(reference=w503, "DisabledEnum"=T7."Disabled and Grayed Out" ("Disabled")) -> ()  [unwired: 1 in, 2 out]
              }
              frame "Pert" {
                n236 = property on="Mode Knees" class="RadioBtnsControl (strict)"() -> ("Controls[]"=w511:refnum<vi>[])  [unwired: 2 in, 2 out]
                n237 = Index Array(array=w511, index #1=0 ("index"), index #2=1 ("index"), index #3=2 ("index")) -> (element #1=w521:refnum<vi>, element #2=w513:refnum<vi>, element #3=w514:refnum<vi>)
                n238 = property class="Ctl"(reference=w521, "DisabledEnum"=T7."Disabled and Grayed Out" ("Disabled")) -> ()  [unwired: 1 in, 2 out]
                n239 = property class="Ctl"(reference=w513, "DisabledEnum"=T7."Enabled" ("Disabled")) -> ()  [unwired: 1 in, 2 out]
                n240 = property class="Ctl"(reference=w514, "DisabledEnum"=T7."Disabled and Grayed Out" ("Disabled")) -> ()  [unwired: 1 in, 2 out]
              }
            }
            n241 = shared-variable "NI-PXIe8880-2F170198\\variables_AlwaysInUse - networkPublished.lvlib\\Mode_knees"(w478) -> ()  [unwired: 1 in, 1 out]
          }
          event "UseVicon": Value Change {
            n242 = event-data() -> ("NewVal"=w522:bool)  [unwired: 1 in, 5 out]
            n243 = Select(t=enum32{"Vicon", "no Vicon"}."Vicon", s=w522, f=enum32{"Vicon", "no Vicon"}."no Vicon") -> (s? t:f=→"ViconTab":enum32{"Vicon", "no Vicon"})
          }
          event "Connect\nVicon": Value Change {
            n244 = event-data() -> ()  [unwired: 1 in, 6 out]
            n245 = call "ConnectVicon.vi"("Mode"="Stream Mode") -> ("error out"=w535:errorcluster, "Connected"=→"Vicon Connected":bool, ".NET Refnum out"=w526:refnum<k24>)  [unwired: 8 in]
            n246 = disable-structure shown="Disabled" {
              frame Disabled {
                w545 = "."
                n247 = invoke class="Client" method="GetVersion"() -> ("GetVersion"=w550:refnum<k24>)  [unwired: 3 in, 2 out]
                n248 = property class="Output_GetVersion"(reference=w550) -> (reference out=w541:refnum<k24>, "Major"=w549:u32, "Minor"=w547:u32, "Point"=w548:u32)  [unwired: 1 in, 1 out]
                n249 = Close Reference(reference=w541) -> ()  [unwired: 1 in, 1 out]
                n250 = Number To Decimal String(number=w549) -> (decimal integer string=w546:string)  [unwired: 1 in]
                n251 = Number To Decimal String(number=w547) -> (decimal integer string=w543:string)  [unwired: 1 in]
                n252 = Number To Decimal String(number=w548) -> (decimal integer string=w544:string)  [unwired: 1 in]
                n253 = Concatenate Strings(w546, w545, w543, w545, w544) -> (→"SDK Version":string)
              }
              frame Enabled {
              }
            }
            n254 = invoke class="Client" method="GetFrame"(reference=w526, error in=w535) -> (reference out=w532:refnum<k24>, error out=w531:errorcluster)  [unwired: 1 in, 1 out]
            n255 = call "FrameNo.vi"("error in (no error)"=w531, ".NET Refnum in"=w532) -> ("error out"=w529:errorcluster, "FrameNumber"=w528:dbl, ".NET Reference out"=w530:refnum<k24>)  [unwired: 7 in]
            n256 = To Double Precision Float(number=w528) -> (double precision float=→"Frame Number":dbl)
            n257 = call "SubName.vi"("error in (no error)"=w529, ".NET Refnum in"=w530) -> ("error out"=w538:errorcluster, "SubjectName"=w536:string, ".NET Refnum out"=w533:refnum<k24>)  [unwired: 7 in]
            "Subject Name" <- w536
            n258 = call "Markers.vi"("error in (no error)"=w538, "Subject Name"=w536, ".NET Refnum in"=w533) -> ("Markers Count"=→"Markers Count":u32, ".NET Reference out"=→".NET Reference out":refnum<k24>)  [unwired: 5 in, 2 out]
          }
          event "Update\nMarkers": Value Change {
            n259 = event-data() -> ()  [unwired: 1 in, 6 out]
          }
          event "Vicon Static": Value Change {
            n260 = event-data() -> ()  [unwired: 1 in, 6 out]
          }
          event "Update Pert Parameters": Value Change {
            # "These are the Pert Parameters"
            n261 = event-data() -> ()  [unwired: 1 in, 6 out]
            n262 = shared-variable "NI-PXIe8880-2F170198\\Perturbation.lvlib\\Pert Direction"("Pert Direction") -> ()  [unwired: 1 in, 1 out]
            n263 = Multiply(x="Weight [Kg]", y=2.20462262) -> (x*y=→"Weight [lbs]":dbl)
            n264 = Divide(x="Amp [%BW]", y=100.0) -> (x/y=w557:dbl)
            n265 = Multiply(x="Weight [Kg]", y=9.98) -> (x*y=w556:dbl)
            n266 = Multiply(x=w557, y=w556) -> (x*y=w552:dbl)
            n267 = Build Array("Rise Time", "Constant Time", "Fall Time", w552) -> (w551:dbl[])
            n268 = shared-variable "NI-PXIe8880-2F170198\\Perturbation.lvlib\\Pert Param"(w551) -> ()  [unwired: 1 in, 1 out]
          }
          event "Update Pert Parameters 2": Value Change {
            n269 = event-data() -> ()  [unwired: 1 in, 6 out]
            n270 = shared-variable "NI-PXIe8880-2F170198\\Perturbation.lvlib\\Pert Direction_pel"("Pert Direction 2") -> ()  [unwired: 1 in, 1 out]
            n271 = Multiply(x="Weight [Kg] 3", y=2.20462262) -> (x*y=→"Weight [lbs] 3":dbl)
            n272 = Divide(x="Amp [%BW] 3", y=100.0) -> (x/y=w575:dbl)
            n273 = Multiply(x="Weight [Kg] 3", y=9.98) -> (x*y=w574:dbl)
            n274 = Multiply(x=w575, y=w574) -> (x*y=w573:dbl)
            n275 = Build Array("Rise Time 2", "Constant Time 2", "Fall Time 2", w573) -> (w566:dbl[])
            n276 = shared-variable "NI-PXIe8880-2F170198\\Perturbation.lvlib\\Pert Param 2"(w566) -> ()  [unwired: 1 in, 1 out]
          }
          event "Apply Pert": Value Change {
            n277 = event-data() -> ()  [unwired: 1 in, 6 out]
            n278 = shared-variable "NI-PXIe8880-2F170198\\ForceField.lvlib\\Apply Pert"("Apply Pert") -> ()  [unwired: 1 in, 1 out]
          }
          event "Apply Pert 2": Value Change {
            n279 = event-data() -> ()  [unwired: 1 in, 6 out]
            n280 = shared-variable "NI-PXIe8880-2F170198\\ForceField.lvlib\\Apply Pert_pel"("Apply Pert 2") -> ()  [unwired: 1 in, 1 out]
          }
          event "Refresh Center": Value Change {
            # "need to test"
            n281 = event-data() -> ()  [unwired: 1 in, 6 out]
            n282 = local read "trunk markers"() -> (w582:dbl[])
            n283 = shared-variable "NI-PXIe8880-2F170198\\ForceField.lvlib\\Refresh Center"("Refresh Center") -> ()  [unwired: 1 in, 1 out]
            n284 = call "getCenterpt.vi"("markers3"=w582) -> ("centerxyz"=w581:dbl[])  [unwired: 3 in]
            n285 = shared-variable "NI-PXIe8880-2F170198\\ForceField.lvlib\\trunk_cn"(w581) -> ()  [unwired: 1 in, 1 out]
          }
          event "Refresh Center 2": Value Change {
            n286 = event-data() -> ()  [unwired: 1 in, 6 out]
            n287 = flat-sequence {
              tunnel: [w587] -> w585
              tunnel: ["Refresh Center 2"] -> w584
              tunnel: w585 -> [w590]
              tunnel: w584 -> [w589]
              frame #0 {
                n288 = local read "pel markers"() -> (w588:dbl[])
                n289 = call "getCenterpt_pel.vi"("markers4"=w588) -> ("centerxyz"=w587:dbl[])  [unwired: 3 in]
              }
              frame #1 {
                n290 = shared-variable "NI-PXIe8880-2F170198\\ForceField.lvlib\\pel_cn"(w590) -> ()  [unwired: 1 in, 1 out]
                n291 = shared-variable "NI-PXIe8880-2F170198\\ForceField.lvlib\\Refresh Center_pel"(w589) -> ()  [unwired: 1 in, 1 out]
              }
            }
          }
          event "Pert Reset": Value Change {
            n292 = event-data() -> ()  [unwired: 1 in, 6 out]
            n293 = shared-variable "NI-PXIe8880-2F170198\\ForceField.lvlib\\Pert Reset"("Pert Reset") -> ()  [unwired: 1 in, 1 out]
          }
          event "Pert Reset 2": Value Change {
            n294 = event-data() -> ()  [unwired: 1 in, 6 out]
            n295 = shared-variable "NI-PXIe8880-2F170198\\ForceField.lvlib\\Pert Reset_pel"("Pert Reset 2") -> ()  [unwired: 1 in, 1 out]
          }
          event "Update R or FF": Value Change {
            n296 = event-data() -> ()  [unwired: 1 in, 6 out]
            n297 = shared-variable "NI-PXIe8880-2F170198\\ForceField.lvlib\\Radius"("Force Field Radius (m)") -> ()  [unwired: 1 in, 1 out]
            n298 = shared-variable "NI-PXIe8880-2F170198\\ForceField.lvlib\\Radius_Update"("Update R or FF") -> ()  [unwired: 1 in, 1 out]
            n299 = shared-variable "NI-PXIe8880-2F170198\\ForceField.lvlib\\FM --- FF"("FM --- FF") -> ()  [unwired: 1 in, 1 out]
            n300 = call "File Dialog"("start path"="Select File with Trunk\nBoundary Points") -> ("selected path"=w599:path)  [unwired: 11 in, 3 out]
            n301 = call-poly <vilib>:"Read Delimited Spreadsheet.vi"("file path (dialog if empty)"=w599, "delimiter (\\t)"="," ("delimiter (\\t)")) -> ("all rows"=w597:dbl[][])  [unwired: 8 in, 5 out]
            n302 = Index Array(array=w597, index (col)=0 ("disabled index (col)")) -> (element=w595:dbl[])  [unwired: 1 in]
            n303 = Index Array(array=w597, index (col)=1 ("disabled index (col)")) -> (element=w593:dbl[])  [unwired: 1 in]
            n304 = shared-variable "NI-PXIe8880-2F170198\\ForceField.lvlib\\Boundary X pts"(w595) -> ()  [unwired: 1 in, 1 out]
            n305 = shared-variable "NI-PXIe8880-2F170198\\ForceField.lvlib\\Boundary Y pts"(w593) -> ()  [unwired: 1 in, 1 out]
          }
          event "Update R or FF 2": Value Change {
            n306 = event-data() -> ()  [unwired: 1 in, 6 out]
            n307 = shared-variable "NI-PXIe8880-2F170198\\ForceField.lvlib\\FM --- FF_pel"("FM --- FF 2") -> ()  [unwired: 1 in, 1 out]
            n308 = shared-variable "NI-PXIe8880-2F170198\\ForceField.lvlib\\Radius_pel"("Pelvis Radius FF") -> ()  [unwired: 1 in, 1 out]
            n309 = shared-variable "NI-PXIe8880-2F170198\\ForceField.lvlib\\Radius_Update_pel"("Update R or FF 2") -> ()  [unwired: 1 in, 1 out]
            n310 = Divide(x="% Body Weight 2", y=100.0) -> (x/y=w612:dbl)
            n311 = Multiply(x="Weight (Kg) --- FF 2", y=9.81) -> (x*y=w609:dbl)
            n312 = Multiply(x=w609, y=w612) -> (x*y=w604:dbl)
            n313 = shared-variable "NI-PXIe8880-2F170198\\ForceField.lvlib\\K constant_pel"(w604) -> ()  [unwired: 1 in, 1 out]
          }
          event "record trajectory": Value Change {
            n314 = event-data() -> ()  [unwired: 1 in, 6 out]
          }
          event "Reset Label": Value Change {
            n315 = event-data() -> ()  [unwired: 1 in, 6 out]
            n316 = shared-variable "NI-PXIe8880-2F170198\\ForceField.lvlib\\downorUp"(FALSE) -> ()  [unwired: 1 in, 1 out]
          }
          event "Update_setForces": Value Change {
            n317 = event-data() -> ()  [unwired: 1 in, 6 out]
            n318 = shared-variable "NI-PXIe8880-2F170198\\ForceField.lvlib\\3D FF Parameters"("Set Unit Force Vector") -> ()  [unwired: 1 in, 1 out]
            n319 = Divide "kg"(x="Weight (lb)", y=2.205) -> (x/y=w623:dbl)
            n320 = Divide(x="Set % Body Weight", y=100.0) -> (x/y=w619:dbl)
            n321 = Multiply(x=w623, y=9.81) -> (x*y=w618:dbl)
            n322 = Multiply(x=w619, y=w618) -> (x*y=w617:dbl)
            n323 = shared-variable "NI-PXIe8880-2F170198\\ForceField.lvlib\\K constant_pel"(w617) -> ()  [unwired: 1 in, 1 out]
            n324 = shared-variable "NI-PXIe8880-2F170198\\ForceField.lvlib\\resetPelvicF"("Update_setForces") -> ()  [unwired: 1 in, 1 out]
          }
          event "Use ATI": Value Change {
            # "send to target"
            n325 = event-data() -> ("NewVal"=w626:bool)  [unwired: 1 in, 5 out]
            n326 = shared-variable "NI-PXIe8880-2F170198\\variables_AlwaysInUse - networkPublished.lvlib\\Use ATI"(w626) -> ()  [unwired: 1 in, 1 out]
            n327 = disable-structure shown="Disabled" {
              frame Disabled {
                # "Needs to be run one time as long the sensor is the same.\nIf sensor is changed, run this module ... generate the \nCalbMatrix and create a constant .... copy and paste in \nthe target program."
                n328 = call "ATICalbMatrix.vi"("Automation Refnum in"="ATIDAQFT._FTSensor") -> ()  [unwired: 9 in, 2 out]
              }
              frame Enabled {
              }
            }
          }
          event "ATI Bias": Value Change {
            n329 = event-data() -> ()  [unwired: 1 in, 6 out]
            n330 = shared-variable "NI-PXIe8880-2F170198\\variables_ATI - networkPublished.lvlib\\Bias"("ATI Bias") -> ()  [unwired: 1 in, 1 out]
          }
          event "ATI UnBias": Value Change {
            n331 = event-data() -> ()  [unwired: 1 in, 6 out]
            n332 = shared-variable "NI-PXIe8880-2F170198\\variables_ATI - networkPublished.lvlib\\UnBias"("ATI UnBias") -> ()  [unwired: 1 in, 1 out]
          }
          event "DataSave": Value Change {
            n333 = event-data() -> ("NewVal"=w630:bool)  [unwired: 1 in, 5 out]
            n334 = flat-sequence {
              tunnel: [w636] -> w631
              tunnel: w630 -> [w636]
              tunnel: w631 -> [w638]
              frame #0 {
                n335 = local read "Subject Name"() -> (w635:string)
                n336 = Concatenate Strings(w635, "_" ("string"), "Insert Test Name", ".txt" ("string")) -> (w637:string)
                "Current Filename" <- w637
                n337 = shared-variable "NI-PXIe8880-2F170198\\variables_SaveData - networkPublished.lvlib\\FileName"(w637) -> ()  [unwired: 1 in, 1 out]
              }
              frame #1 {
                n338 = shared-variable "NI-PXIe8880-2F170198\\variables_SaveData - networkPublished.lvlib\\SaveData"(w638) -> ()  [unwired: 1 in, 1 out]
              }
            }
          }
        }
      }
      n339 = node-c288(i64 10 ("Period"), 60000 ("Priority")) -> (w35:T8)  [unwired: 2 in]
      n340 = timed-loop {
        timing: w35 -> [_]
        timing-out: [_] -> w34
        stop <- w145 stop-if-true
        # "If (use cond.) TCP is valid, \nADD code to \ncheck to see if TCP\nis still valid. If not, change\nthe value. This will make code \ntry to reconnect when it drops"
        n341 = node-c288() -> (→"Finished Late? [i-1]":bool)  [unwired: 1 in, 3 out]
        n342 = local read "TCP connection to Unity?"() -> (w144:bool)
        n343 = case shown="False" w144 {
          frame False {
            n344 = local read "Control point data source"() -> (w149:T2)
            n345 = case shown="\"Unity\"" w149 {
              frame "None/Off", Default {
              }
              frame "Vicon" {
              }
              frame "Unity" {
                w154 = u16 8052 ("remote port or service name")
                w153 = "localhost" ("address")
                # "If not connected, keep updating the \nbase value for when the last message was \nreceived, so it is accurate when a \nconnection is made."
                n346 = TCP Open Connection(address=w153, remote port or service name=w154, error in (no error)=errorcluster {"status"=FALSE, "code"=0, "source"=""}) -> (connection ID=→"Unity TCP connection ID":refnum<k5>, error out=w151:errorcluster)  [unwired: 2 in]
                n347 = TCP Create Listener(8:w151, 10:w154, 11:w153) -> (0:w150:errorcluster, 3:→"listener ID":refnum<k5>)  [unwired: 2 in, 1 out]
                n348 = case shown="No Error" w150 {
                  frame No Error {
                    n349 = local write "TCP connection to Unity?"(TRUE ("TCP connection to Unity?")) -> ()
                  }
                  frame Error {
                    # "TCP connection to Unity failed\n (perhaps a timeout or bad IP)"
                  }
                }
                n350 = Tick Count (ms)() -> (millisecond timer value=w155:u32)
                n351 = local write "LastTimeUnityTensionsReceivedInMs"(w155) -> ()
              }
            }
          }
          frame True {
            n352 = flat-sequence {
              frame #0 {
                n353 = case shown="\"Unity\"" "Control point data source" {
                  frame "None/Off", Default {
                  }
                  frame "Vicon" {
                  }
                  frame "Unity" {
                    # "Read a single ASCII message terminated with the \nCRLF character. Note: this will NOT flush the \nbuffer, as it only reads a single ASCII message."
                    # "Tokenize received \nstring"
                    n354 = local read "Unity TCP connection ID"() -> (w171:refnum<k5>)
                    n355 = TCP Read(connection ID=w171, bytes to read=1000, 7:T11."CRLF" ("mode (standard)"), 9:75 ("timeout ms (25000)")) -> (data out=w170:string)  [unwired: 1 in, 2 out]
                    n356 = call "Tokenize string on commas.vi"("Unity TCP data received"=w170) -> ("Tokenized Unity Message"=w172:string[])  [unwired: 10 in]
                    "Tokenized Unity Message" <- w172
                    n357 = call "Parse_TCP_Message_From_Unity.vi"("Tokenized message string array"=w172) -> ("task Over Message Received Flag"=w160:bool, "Desired tensions by motor"=w163:T12, "Control point position coords"=w169:dbl[], "Command string"=w168:string, "Force field type specifier"=w165:string, "Center point of FF"=w167:dbl[], "File information string"=w161:string, "Trunk Structure Matrix"=w164:dbl[][], "Boundary points"=w166:dbl[])  [unwired: 6 in]
                    n358 = case shown="\"O\"" w168 {
                      tunnel: w169 -> [_ w176 _ _ _ _ _ _ _]
                      tunnel: w167 -> [_ _ w178 _ _ _ _ _ _]
                      tunnel: w166 -> [_ _ _ _ w182 _ _ _ _]
                      tunnel: w165 -> [_ _ _ w180 _ _ _ _ _]
                      tunnel: w164 -> [_ _ _ _ _ w185 _ _ _]
                      tunnel: w163 -> [_ _ _ _ _ _ w188 _ _]
                      tunnel: w161 -> [_ _ _ _ _ _ _ w216 _]
                      tunnel: w160 -> [_ _ _ _ _ _ _ _ w217]
                      frame "", Default {
                      }
                      frame "C" {
                        n359 = shared-variable "NI-PXIe8880-2F170198\\variables_Unity_Data.lvlib\\FF Control Point"(w176) -> (error out=w175:errorcluster)  [unwired: 1 in]
                        n360 = call <vilib>:"Flush Shared Variable Data.vi"("error in (no error)"=w175) -> ()  [unwired: 10 in, 1 out]
                        "Control point position coords" <- w176
                      }
                      frame "O" {
                        n361 = shared-variable "NI-PXIe8880-2F170198\\variables_Unity_Data.lvlib\\Center Point for FF"(w178) -> (error out=w177:errorcluster)  [unwired: 1 in]
                        n362 = call <vilib>:"Flush Shared Variable Data.vi"("error in (no error)"=w177) -> ()  [unwired: 10 in, 1 out]
                        "Center point for FF" <- w178
                      }
                      frame "F" {
                        # "Assign the force field type specifier string to the \nfront-panel display (for viewing) and to the \nnetwork-published var (for sending to PXI)"
                        n363 = shared-variable "NI-PXIe8880-2F170198\\variables_Unity_Data.lvlib\\Force Field Type Specifier"(w180) -> (error out=w179:errorcluster)  [unwired: 1 in]
                        n364 = call <vilib>:"Flush Shared Variable Data.vi"("error in (no error)"=w179) -> ()  [unwired: 10 in, 1 out]
                        "Trunk FF type specifier" <- w180
                      }
                      frame "E" {
                        n365 = shared-variable "NI-PXIe8880-2F170198\\variables_Unity_Data.lvlib\\Excursion Distances Vicon Frame"(w182) -> (error out=w181:errorcluster)  [unwired: 1 in]
                        n366 = call <vilib>:"Flush Shared Variable Data.vi"("error in (no error)"=w181) -> ()  [unwired: 10 in, 1 out]
                        "Excursion distances Vicon frame" <- w182
                      }
                      frame "T" {
                        # "We pass the S matrix as a 1D array, since we\ncannot use 2D arrays as network-published \nvariables. NOTE: since we must specify the \nnumber of elements, this is our current limitation\non flexibly choosing the number of motors per belt."
                        n367 = Reshape Array(w185, 24 ("dimension size")) -> (w184:dbl[])
                        n368 = shared-variable "NI-PXIe8880-2F170198\\variables_Unity_Data.lvlib\\Trunk Structure Matrix"(w184) -> (error out=w183:errorcluster)  [unwired: 1 in]
                        n369 = call <vilib>:"Flush Shared Variable Data.vi"("error in (no error)"=w183) -> ()  [unwired: 10 in, 1 out]
                        "Trunk Structure Matrix" <- w185
                      }
                      frame "K" {
                        n370 = flat-sequence {
                          tunnel: w188 -> [w201]
                          tunnel: [w191] -> w187
                          tunnel: w187 -> [w214]
                          frame #0 {
                            # "\"K\" is the primary update tensions command. \nMost other messages are no longer used. \nOther still-used message headers: \n\"I\" = information (about subject, date, time)"
                            # "In for loop, we subtract 1 \nfrom motor index because\nLabview is zero-indexed."
                            # "Motors for which a desired tension value were sent \nare put into the array at their corresponding index. \nMotors without specified tension values are set to 0.\nResult = an ordered array (motors 1-14) with desired tensions."
                            n371 = Unbundle By Name(w201) -> ("Most Recent Vicon Frame Number"=w190:u32, "Corresponding motor tensions"=w198:dbl[], "Motor numbers"=w200:i32[])
                            "Last Vicon Frame Read" <- w190
                            n372 = Initialize Array(0.0 ("element"), "Total Number Motors") -> (w199:dbl[])
                            n373 = for {
                              tunnel: w200 -> [w206] mode=indexing
                              shift-right: [w207] -> w197
                              shift-left: w199 -> [w209]
                              tunnel: w198 -> [w208] mode=indexing
                              n374 = Subtract(x=w206, y=1) -> (x-y=w204:i32)
                              n375 = Replace Array Subset(array=w209, new element=w208, index=w204) -> (w207:dbl[])
                            }
                            "UnityDesiredCableTensionsInAscendingOrder" <- w197
                            n376 = shared-variable "NI-PXIe8880-2F170198\\variables_Unity_Data.lvlib\\MostRecentViconFrameNumber"(w190) -> ()  [unwired: 1 in, 1 out]
                            n377 = local read "LastTimeUnityTensionsReceivedInMs"() -> (w196:u32)
                            n378 = Tick Count (ms)() -> (millisecond timer value=w191:u32)
                            n379 = Subtract(x=w191, y=w196) -> (x-y=w195:u32)
                            n380 = Divide(x=w195, y=u32 1000) -> (x/y=w193:dbl)
                            n381 = Divide(x=1.0, y=w193) -> (x/y=→"TensionsUpdateRateHz":dbl)
                          }
                          frame #1 {
                            # "Flush the TCP buffer by reading a \nlarge amount of bytes in \nStandard Mode."
                            # "This frame is needed (ugh) to track\nthe update rate for receiving the \n\"K\" (update tensions) command."
                            n382 = local read "Unity TCP connection ID"() -> (w210:refnum<k5>)
                            n383 = TCP Read(connection ID=w210, bytes to read=500, 7:T11."Standard" ("mode (standard)"), 9:1 ("timeout ms (25000)")) -> ()  [unwired: 1 in, 3 out]
                            "LastTimeUnityTensionsReceivedInMs" <- w214
                          }
                        }
                      }
                      frame "I" {
                        "Unity task info string" <- w216
                        "New info string received" <- TRUE ("New info string received")
                      }
                      frame "S" {
                        "Task has ended flag" <- w217
                      }
                    }
                  }
                }
              }
            }
          }
        }
        n384 = node-c288() -> ()  [unwired: 1 in, 1 out]
        n385 = local read "Stop"() -> (w145:bool)
      }
      n386 = node-c288(w37) -> ()  [unwired: 1 out]
      n387 = node-c288(i64 10 ("Period"), 1 ("Priority")) -> (w28:T8)  [unwired: 7 in]
      n388 = timed-loop {
        timing: w28 -> [_]
        timing-out: [_] -> w27
        stop <- w39 stop-if-true
        n389 = node-c288() -> ()  [unwired: 1 in, 1 out]
        n390 = flat-sequence {
          tunnel: [w75] -> w39
          frame #0 {
            # "For each column, which is \nthe history for one sensor."
            # "Compute and store tension sensor \nstandard deviation."
            # "Below: store tension history\nin a local variable and compute \nstandard deviation of tension \nsensor history."
            # "We record only when we are connected to Unity."
            n391 = shared-variable "NI-PXIe8880-2F170198\\variables_Unity_Data.lvlib\\DesiredTensionsInAscendingMotorOrder"() -> (w60:dbl[])  [unwired: 1 in, 1 out]
            n392 = local read "All tensions history"() -> (w52:dbl[][])
            n393 = local read "Unity task info string"() -> (w67:string)
            n394 = local read "Task has ended flag"() -> (w61:bool)
            n395 = local read "New info string received"() -> (w65:bool)
            n396 = Array Size(array=w52) -> (size(s)=w54:i32[])
            n397 = local read "Connected to Unity last save call?"() -> (w63:bool)
            n398 = shared-variable "NI-PXIe8880-2F170198\\variables_Unity_Data.lvlib\\AllCurrentTensions"() -> (w49:dbl[])  [unwired: 1 in, 1 out]
            n399 = Index Array(array=w54, index=1) -> (element=w45:i32)
            n400 = Index Array(array=w54, index=0) -> (element=w47:i32)
            n401 = local read "Last Vicon Frame Read"() -> (w66:u32)
            n402 = local read "TCP connection to Unity?"() -> (w74:bool)
            n403 = Subtract(x=w47, y=1.0) -> (x-y=w56:dbl)
            n404 = local read "Current save file out"() -> (w71:path)
            n405 = Array Subset(array=w52, index (row)=0 ("index"), length (row)=w56, index (col)=0 ("index"), length (col)=w45) -> (w51:dbl[][])
            n406 = local read "Data to save"() -> (w68:dbl[][])
            n407 = call "write_markerdata.vi"("Data to save in"=w68, "Connected to Unity last call? In"=w63, "Connected to Unity via TCP?"=w74, "Host folder"=path "C:/Users/ROAR/Documents/Rob Motor Assessment stuff/Labview/RobUST_3D_with_Unity_Control_PXI_Low_Level_Only_Streamlined/Recorded_Data", "Unity task info string"=w67, "DesiredTensions"=w60, "Current save file in"=w71, "CurrentTensions"=w49, "New task info string flag in"=w65, "Last Vicon frame read"=w66, "Task has ended flag"=w61) -> ("Connected to Unity last call? Out"=→"Connected to Unity last save call?":bool, "Current save file out"=→"Current save file out":path, "Data to save"=→"Data to save":dbl[][], "New task info string flag out"=w64:bool, "Task had ended flag out"=w62:bool)  [unwired: 4 in]
            n408 = local read "Stop"() -> (w75:bool)
            n409 = Insert Into Array(array=w51, index (row)=0, new element=w49) -> (w48:dbl[][])  [unwired: 1 in]
            n410 = local write "New info string received"(w64) -> ()
            n411 = local write "All tensions history"(w48) -> ()
            n412 = local read "All tensions standard dev"() -> (w46:dbl[])
            n413 = local read "All tensions mean"() -> (w43:dbl[])
            n414 = local write "Task has ended flag"(w62) -> ()
            n415 = for {
              N: w45 -> [_]
              shift-right: [w80] -> _
              shift-left: w48 -> [w80]
              tunnel: w45 -> [_]
              shift-right: [w81] -> w44
              shift-left: w46 -> [w83]
              shift-right: [w76] -> w42
              shift-left: w43 -> [w77]
              i -> [w79]
              n416 = Index Array(array=w80, index (col)=w79) -> (element=w84:dbl[])  [unwired: 1 in]
              n417 = call <vilib>:"Std Deviation and Variance.vi"("X"=w84) -> ("mean"=w78:dbl, "standard deviation"=w82:dbl)  [unwired: 1 in, 1 out]
              n418 = Replace Array Subset(array=w77, new element=w78, index=w79) -> (w76:dbl[])
              n419 = Replace Array Subset(array=w83, new element=w82, index=w79) -> (w81:dbl[])
            }
            "All tensions mean" <- w42
            n420 = local write "All tensions standard dev"(w44) -> ()
          }
          frame #1 {
            n421 = Wait (ms)(milliseconds to wait=u32 20) -> ()  [unwired: 1 out]
          }
        }
        n422 = node-c288() -> ()  [unwired: 1 in, 1 out]
      }
      n423 = node-c288(w27) -> ()  [unwired: 1 out]
      n424 = node-c288(i64 5 ("Period")) -> (w31:T8)  [unwired: 3 in]
      n425 = timed-loop {
        timing: w31 -> [_]
        timing-out: [_] -> w30
        stop <- _ stop-if-true
        # "The only way to reliably check if a TCP connection\nis still open is to see the last time we got data. If it \nhas been more than 50 ms since we received a \"K\"\ncommand, close the TCP connection."
        n426 = node-c288() -> ()  [unwired: 1 in, 1 out]
        n427 = local read "LastTimeUnityTensionsReceivedInMs"() -> (w133:u32)
        n428 = Tick Count (ms)() -> (millisecond timer value=w134:u32)
        n429 = Subtract(x=w134, y=w133) -> (x-y=w132:u32)
        n430 = Greater?(x=w132, y=u32 3000) -> (0:w130:bool)
        n431 = case shown="True" w130 {
          frame False {
          }
          frame True {
            n432 = local read "Unity TCP connection ID"() -> (w135:refnum<k5>)
            n433 = local write "TCP connection to Unity?"(FALSE ("TCP connection to Unity?")) -> ()
            n434 = TCP Close Connection(connection ID=w135) -> ()  [unwired: 2 in, 2 out]
          }
        }
        n435 = node-c288() -> ()  [unwired: 1 in, 1 out]
      }
      n436 = node-c288(w34) -> ()  [unwired: 1 out]
      n437 = node-c288(w30) -> ()  [unwired: 1 out]
    }
  }
